vi "MPU_Stick_UI_Event_Handler.vi"(8 "error in (no error)":errorcluster, 11 "MPU_Stick_Globals":T3) -> ()   [LabVIEW 2017]
uses:
  Controls/MPU_Stick_Globals.ctl
  Controls/IMU_Configuration_References.ctl
  Controls/MP_Comp_Filter_Constants_References.ctl
  Controls/MD_Threshold_References.ctl
  Controls/MD_Type_References.ctl
  Controls/LED_Configuration_References.ctl
  Controls/Primary_References.ctl
  Controls/MPU_Stick_Queues.ctl
  Controls/MPU_Stick_Queue_Element.ctl
  Controls/MPU_Stick_Queue_Commands.ctl
  Classes/ADCP.lvclass
  <vilib>/Utility/miscctls.llb/LVPointDoubleTypeDef.ctl
  Controls/MPU_Stick_Read_Write_Configurations_Command.ctl
  Controls/MPU_Stick_Config_Parameters.ctl
  Controls/MPU_Stick_Plotter_Core_Commands.ctl
  <vilib>/Utility/miscctls.llb/LVOffsetAndMultiplierTypeDef.ctl
  MPU_Stick_Read_Serial_Port_Emulator.vi
panel:
  out "Primary.Parameter to monitor A":T1(ring)
  out "Primary.Cursor Position":T2
  out "Primary.Parameter to monitor":T1(ring)
  out "Primary.Offset":dbl
  out "Primary.Gain":dbl
  out "Primary.Get Gain & Offset":bool
  out "Primary.Set Gain & Offset":bool
  out "Primary.Remove graph parameter":bool
  out "Primary.Add graph parameter":bool
  out "MD Types Config.Set Parameter Index":u32
  out "MD Types Config.Get Parameter Index":u32
  out "MD Thresholds Config.Get Parameter Index":u32
  out "MD Thresholds Config.Set Parameter Index":u32
  out "Filter constants Config.Set Parameter Index":u32
  out "Filter constants Config.Get Parameter Index":u32
  out "LED Config.Set Parameter Index":u32
  out "LED Config.Get Parameter Index":u32
  out "IMU Config.Set Parameter Index":u32
  out "IMU Config.Get Parameter Index":u32
  out "Primary.MP Reset":bool
  out "Primary.Calibrate Sensor":bool
  out "Primary.Save all config":bool
  out "Primary.Write all config":bool
  out "Primary.Read all config":bool
  out "Primary.Connect Device":bool
  out "Primary.Exit Application":bool
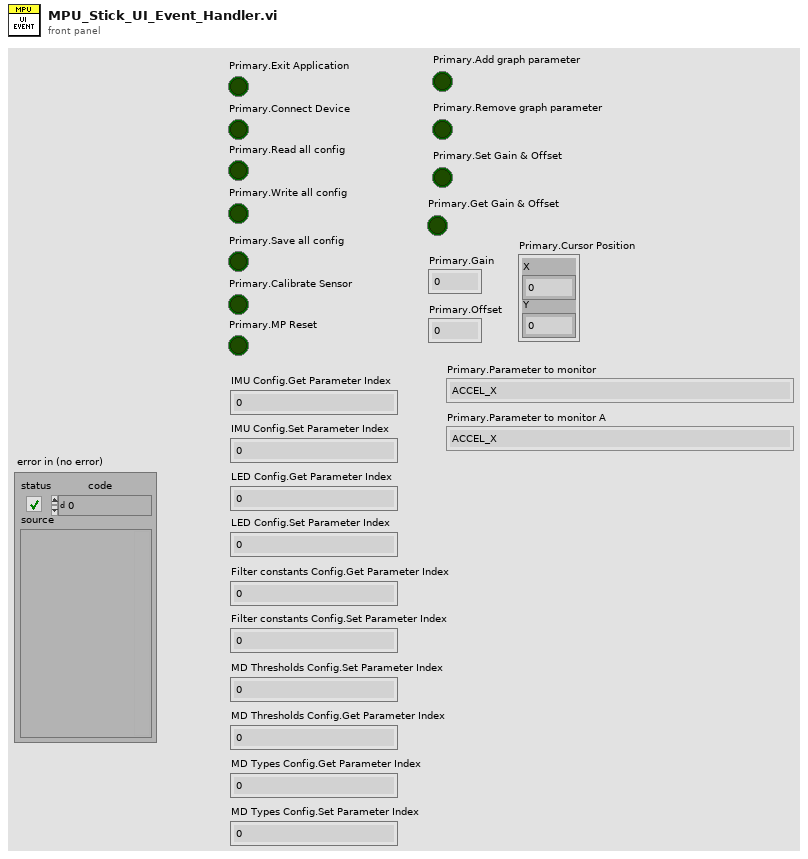
[diagram p1: front panel]
types:
  T1 = enum16{"ACCEL_X", "ACCEL_Y", "ACCEL_Z", "GYRO_X", "GYRO_Y", "GYRO_Z", "ROLL_ACCEL", "ROLL_GYRO", "ROLL_COMP_FILTER", "PITCH_ACCEL", "PITCH_GYRO", "PITCH_COMP_FILTER", "YAW_ACCEL", "YAW_GYRO", "YAW_COMP_FILTER"}
  T2 = typedef "LVPointDoubleTypeDef.ctl" = cluster{"X":dbl, "Y":dbl}
  T3 = typedef "MPU_Stick_Globals.ctl" = cluster{"IMU_configuration_references":T4, "MP_Comp_Filter_Constants_References":T5, "MD_Threshold_References":T6, "MD_Type_References":T7, "LED_Configuration_References":T8, "Primary_references":T9, "MPU_Stick_Queues":T10, "ADCP":refnum<vi>}
  T4 = typedef "IMU_Configuration_References.ctl" = cluster{"Get all IMU configurations":refnum<vi>, "Set all IMU configurations":refnum<vi>, "Get sampling frequency":refnum<vi>, "Set sampling frequency":refnum<vi>, "Get calibration point count":refnum<vi>, "Set calibration point count":refnum<vi>, "Get calibration interval":refnum<vi>, "Set calibration interval":refnum<vi>, "Get Gyroscope bandwidth":refnum<vi>, "Set Gyroscope bandwidth":refnum<vi>, "Get Gyroscope F.S. Value":refnum<vi>, "Set Gyroscope F.S. Value":refnum<vi>, "Get Accelerometer bandwidth":refnum<vi>, "Set Accelerometer bandwidth":refnum<vi>, "Get Accelerometer F.S. Value":refnum<vi>, "Set Accelerometer F.S. Value":refnum<vi>, "Sampling frequency (Hz)":refnum<vi>, "Calibration point count":refnum<vi>, "Calibration interval (ms)":refnum<vi>, "IMU Gyroscope bandwidth":refnum<vi>, "IMU Gyroscope F.S. value":refnum<vi>, "IMU Accelerometer bandwidth":refnum<vi>, "IMU Accelerometer F.S. value":refnum<vi>}
  T5 = typedef "MP_Comp_Filter_Constants_References.ctl" = cluster{"Set pitch filter constant":refnum<vi>, "Get pitch filter constant":refnum<vi>, "Set roll filter constant":refnum<vi>, "Get roll filter constant":refnum<vi>, "Pitch filter constant":refnum<vi>, "Roll filter constant":refnum<vi>}
  T6 = typedef "MD_Threshold_References.ctl" = cluster{"Yaw threshold (U)":refnum<vi>, "Yaw threshold (L)":refnum<vi>, "Pitch threshold (U)":refnum<vi>, "Pitch. threshold (L)":refnum<vi>, "Roll threshold (U)":refnum<vi>, "Roll threshold (L)":refnum<vi>, "Z gyro. threshold (U)":refnum<vi>, "Z gyro. threshold (L)":refnum<vi>, "Y gyro. threshold (U)":refnum<vi>, "Y gyro. threshold (L)":refnum<vi>, "X gyro. threshold (U)":refnum<vi>, "X gyro. threshold (L)":refnum<vi>, "Z accel. threshold (U)":refnum<vi>, "Z accel. threshold (L)":refnum<vi>, "Y accel. threshold (U)":refnum<vi>, "Y accel. threshold (L)":refnum<vi>, "X accel. threshold (U)":refnum<vi>, "X accel. threshold (L)":refnum<vi>, "Set all Motion detection threshold configurations":refnum<vi>, "Get yaw threshold (upper)":refnum<vi>, "Get yaw threshold (lower)":refnum<vi>, "Get pitch threshold (upper)":refnum<vi>, "Get pitch threshold (lower)":refnum<vi>, "Get roll threshold (upper)":refnum<vi>, "Get roll threshold (lower)":refnum<vi>, "Get Z gyro threshold (upper)":refnum<vi>, "Get Z gyro threshold (lower)":refnum<vi>, "Get Y gyro threshold (upper)":refnum<vi>, "Get Y gyro threshold (lower)":refnum<vi>, "Get X gyro threshold (upper)":refnum<vi>, "Get X gyro threshold (lower)":refnum<vi>, "Get Z accel threshold (upper)":refnum<vi>, "Get Z accel threshold (lower)":refnum<vi>, "Get Y accel threshold (upper)":refnum<vi>, "Get Y accel threshold (lower)":refnum<vi>, "Get X accel threshold (upper)":refnum<vi>, "Get X accel threshold (lower)":refnum<vi>, "Get all Motion detection threshold configurations":refnum<vi>, "Set yaw threshold (upper)":refnum<vi>, "Set yaw threshold (lower)":refnum<vi>, "Set pitch threshold (upper)":refnum<vi>, "Set pitch threshold (lower)":refnum<vi>, "Set roll threshold (upper)":refnum<vi>, "Set roll threshold (lower)":refnum<vi>, "Set Z gyro threshold (upper)":refnum<vi>, "Set Z gyro threshold (lower)":refnum<vi>, "Set Y gyro threshold (upper)":refnum<vi>, "Set Y gyro threshold (lower)":refnum<vi>, "Set X gyro threshold (upper)":refnum<vi>, "Set X gyro threshold (lower)":refnum<vi>, "Set Z accel threshold (upper)":refnum<vi>, "Set Z accel threshold (lower)":refnum<vi>, "Set Y accel threshold (upper)":refnum<vi>, "Set Y accel threshold (lower)":refnum<vi>, "Set X accel threshold (upper)":refnum<vi>, "Set X accel threshold (lower)":refnum<vi>}
  T7 = typedef "MD_Type_References.ctl" = cluster{"Yaw threshold type":refnum<vi>, "Pitch threshold type":refnum<vi>, "Roll threshold type":refnum<vi>, "Z gyro threshold type":refnum<vi>, "Y gyro threshold type":refnum<vi>, "X gyro threshold type":refnum<vi>, "Z accel threshold type":refnum<vi>, "Y accel threshold type":refnum<vi>, "X accel threshold type":refnum<vi>, "Set all Motion detection type configurations":refnum<vi>, "Get all Motion detection type configurations":refnum<vi>, "Set yaw threshold type":refnum<vi>, "Get yaw threshold type":refnum<vi>, "Set pitch threshold type":refnum<vi>, "Get pitch threshold type":refnum<vi>, "Set roll threshold type":refnum<vi>, "Get roll threshold type":refnum<vi>, "Set Z gyroscope threshold type":refnum<vi>, "Get Z gyroscope threshold type":refnum<vi>, "Set Y gyroscope threshold type":refnum<vi>, "Get Y gyroscope threshold type":refnum<vi>, "Set X gyroscope threshold type":refnum<vi>, "Get X gyroscope threshold type":refnum<vi>, "Set Z accel threshold type":refnum<vi>, "Get Z accel threshold type":refnum<vi>, "Set Y accel threshold type":refnum<vi>, "Get Y accel threshold type":refnum<vi>, "Get X accel threshold type":refnum<vi>, "Set X accel threshold type":refnum<vi>}
  T8 = typedef "LED_Configuration_References.ctl" = cluster{"Get all LED configurations":refnum<vi>, "Set all LED configurations":refnum<vi>, "Get LED3 configuration":refnum<vi>, "Set LED3 configuration":refnum<vi>, "Get LED2 configuration":refnum<vi>, "Set LED2 configuration":refnum<vi>, "Get LED1 configuration":refnum<vi>, "Set LED1 configuration":refnum<vi>, "LED3 Configuration":refnum<vi>, "LED2 Configuration":refnum<vi>, "LED1 Configuration":refnum<vi>}
  T9 = typedef "Primary_References.ctl" = cluster{"3D View Image":refnum<vi>, "Plot":refnum<vi>, "Graph / 3D view tab control":refnum<vi>, "MP Reset":refnum<vi>, "Calibrate IMU":refnum<vi>, "Plot Parameter List":refnum<vi>, "Remove Parameter from Plot":refnum<vi>, "Add Parameter to Plot":refnum<vi>, "Parameter to monitor":refnum<vi>, "Yaw motion detection output":refnum<vi>, "Pitch motion detection output":refnum<vi>, "Roll motion detection output":refnum<vi>, "Z gyro motion detection output":refnum<vi>, "Y gyro motion detection output":refnum<vi>, "X gyro motion detection output":refnum<vi>, "Z accel motion detection output":refnum<vi>, "Y accel motion detection output":refnum<vi>, "X accel motion detection output":refnum<vi>, "Yaw angle (filter) (degrees)":refnum<vi>, "Pitch angle (filter) (degrees)":refnum<vi>, "Roll angle (filter) (degrees)":refnum<vi>, "Yaw angle (gyro) (degrees)":refnum<vi>, "Pitch angle (gyro) (degrees)":refnum<vi>, "Roll angle (gyro) (degrees)":refnum<vi>, "Yaw angle (accel) (degrees)":refnum<vi>, "Pitch angle (accel) (degrees)":refnum<vi>, "Roll angle (accel) (degrees)":refnum<vi>, "Z gyroscope reading (DPS)":refnum<vi>, "Y gyroscope reading (DPS)":refnum<vi>, "X gyroscope reading (DPS)":refnum<vi>, "Z accelerometer reading (G)":refnum<vi>, "Y accelerometer reading (G)":refnum<vi>, "X accelerometer reading (G)":refnum<vi>, "Save all config.":refnum<vi>, "Write all config.":refnum<vi>, "Read all config.":refnum<vi>, "Tab Control":refnum<vi>, "Baud Rate":refnum<vi>, "COM Port":refnum<vi>, "Time (ms)":refnum<vi>, "Value (Units)":refnum<vi>, "Exit Application":refnum<vi>, "Connect Device":refnum<vi>, "Progress Bar":refnum<vi>, "Get Range & Offset":refnum<vi>, "Range":refnum<vi>, "Offset":refnum<vi>, "Set Range & Offset":refnum<vi>, "Parameter name":refnum<vi>, "Plot time (ms)":refnum<vi>, "Plot value":refnum<vi>}
  T10 = typedef "MPU_Stick_Queues.ctl" = cluster{"UI Event Handler":refnum<queue>, "3D View Updater":refnum<queue>, "Plot Updater":refnum<queue>, "Serial Port Reader":refnum<queue>, "UI Indicators Updater":refnum<queue>}
  T11 = typedef "MPU_Stick_Queue_Element.ctl" = cluster{"Data":variant, "Command":T12}
  T12 = typedef "MPU_Stick_Queue_Commands.ctl" = enum16{"UI_Event_Exit_Application_RQST", "UI_Event_Exit_Application_ACK", "UI_Event_Connect_Device_RQST", "UI_Event_Connect_Device_ACK", "UI_Event_Disconnect_Device_RQST", "UI_Event_Disconnect_Device_ACK", "UI_Event_Read_All_Configurations_RQST", "UI_Event_Read_All_Configurations_ACK", "UI_Event_Write_All_Configurations_RQST", "UI_Event_Write_All_Configurations_ACK", "UI_Event_Save_All_Configurations_RQST", "UI_Event_Save_All_Configurations_ACK", "UI_Event_Calibrate_IMU_Sensor_RQST", "UI_Event_Calibrate_IMU_Sensor_ACK", "UI_Event_MP_Reset_RQST", "UI_Event_MP_Reset_ACK", "UI_Event_Get_Config_RQST", "UI_Event_Get_Config_ACK", "UI_Event_Set_Config_RQST", "UI_Event_Set_Config_ACK", "Read_Serial_Port_Data_Pause", "Read_Serial_Port_Data_Pause_ACK", "Read_Serial_Port_Data_Continue", "Read_Serial_Port_Data_Exit", "Plotter_Exit", "Plotter_Update", "Plotter_Add_Channel", "Plotter_Remove_Channel", "3D Viewer Update", "3D Viewer Exit", "UI Indicators Update", "UI Indicators Exit"}
  T13 = typedef "MPU_Stick_Plotter_Core_Commands.ctl" = enum16{"Initialize", "Add Channel", "Remove Channel", "Set Channel Minimum Value", "Set Channel Maximum Value", "Set Offset & Multiplier", "Get Offset & Multiplier", "Update Channel", "Get Cursor Data", "Clear", "Reset"}
  T14 = typedef "LVOffsetAndMultiplierTypeDef.ctl" = cluster{"Offset":dbl, "Multiplier":dbl}
  T15 = typedef "MPU_Stick_Config_Parameters.ctl" = enum16{"IMU_ACCEL_FS", "IMU_ACCEL_BW", "IMU_GYRO_FS", "IMU_GYRO_BW", "IMU_CALIB_INTERVAL", "IMU_CALIB_POINT_COUNT", "IMU_SAMPLING_FREQ", "LED1_CONFIG", "LED2_CONFIG", "LED3_CONFIG", "MP_ROLL_FILTER_CONSTANT", "MP_PITCH_FILTER_CONSTANT", "MP_THRESHOLD_X_ACCEL_LOW", "MP_THRESHOLD_X_ACCEL_HIGH", "MP_THRESHOLD_Y_ACCEL_LOW", "MP_THRESHOLD_Y_ACCEL_HIGH", "MP_THRESHOLD_Z_ACCEL_LOW", "MP_THRESHOLD_Z_ACCEL_HIGH", "MP_THRESHOLD_X_GYRO_LOW", "MP_THRESHOLD_X_GYRO_HIGH", "MP_THRESHOLD_Y_GYRO_LOW", "MP_THRESHOLD_Y_GYRO_HIGH", "MP_THRESHOLD_Z_GYRO_LOW", "MP_THRESHOLD_Z_GYRO_HIGH", "MP_THRESHOLD_ROLL_LOW", "MP_THRESHOLD_ROLL_HIGH", "MP_THRESHOLD_PITCH_LOW", "MP_THRESHOLD_PITCH_HIGH", "MP_THRESHOLD_YAW_LOW", "MP_THRESHOLD_YAW_HIGH", "MP_DETECTION_TYPE_X_ACCEL", "MP_DETECTION_TYPE_Y_ACCEL", "MP_DETECTION_TYPE_Z_ACCEL", "MP_DETECTION_TYPE_X_GYRO", "MP_DETECTION_TYPE_Y_GYRO", "MP_DETECTION_TYPE_Z_GYRO", "MP_DETECTION_TYPE_ROLL", "MP_DETECTION_TYPE_PITCH", "MP_DETECTION_TYPE_YAW"}
  T16 = typedef "MPU_Stick_Plotter_Core_Channel_Data.ctl" = cluster{"Value (original)":dbl[], "Time (ms)":dbl[], "Channel name":string, "Minimum":dbl, "Maximum":dbl, "Offset":dbl, "Range":dbl}
  T17 = cluster{"Symbol File Path":path, "Transmit Log File Path":path, "Receive Log File Path":path, "COM Port":refnum<visa-resource-name>, "Baud rate":u32, "Number of retries":u16, "Retry interval (ms)":u16, "Session start time (ms)":u32, "Current time (ms)":u32, "Serialport timeout (ms)":u32}
  T18 = typedef "MPU_Stick_Read_Write_Configurations_Command.ctl" = enum16{"Read", "Write", "Write All", "Read All"}
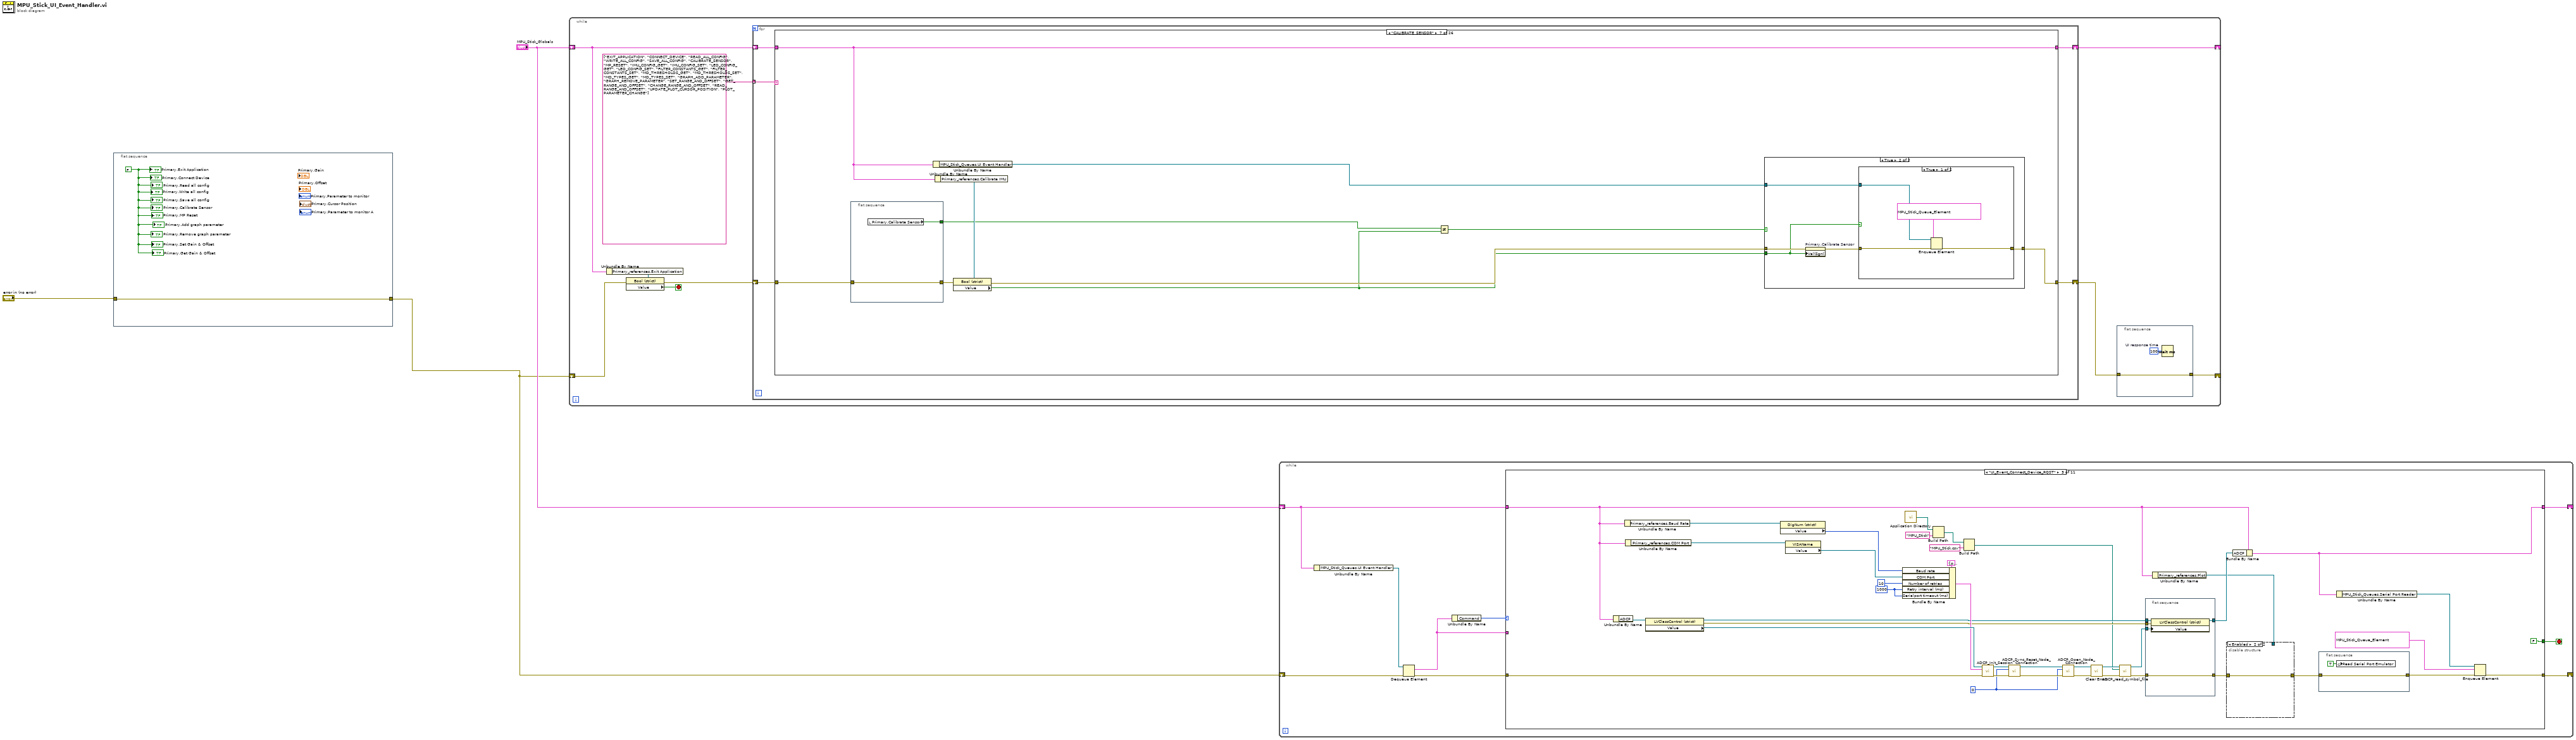
[diagram p0: block diagram]
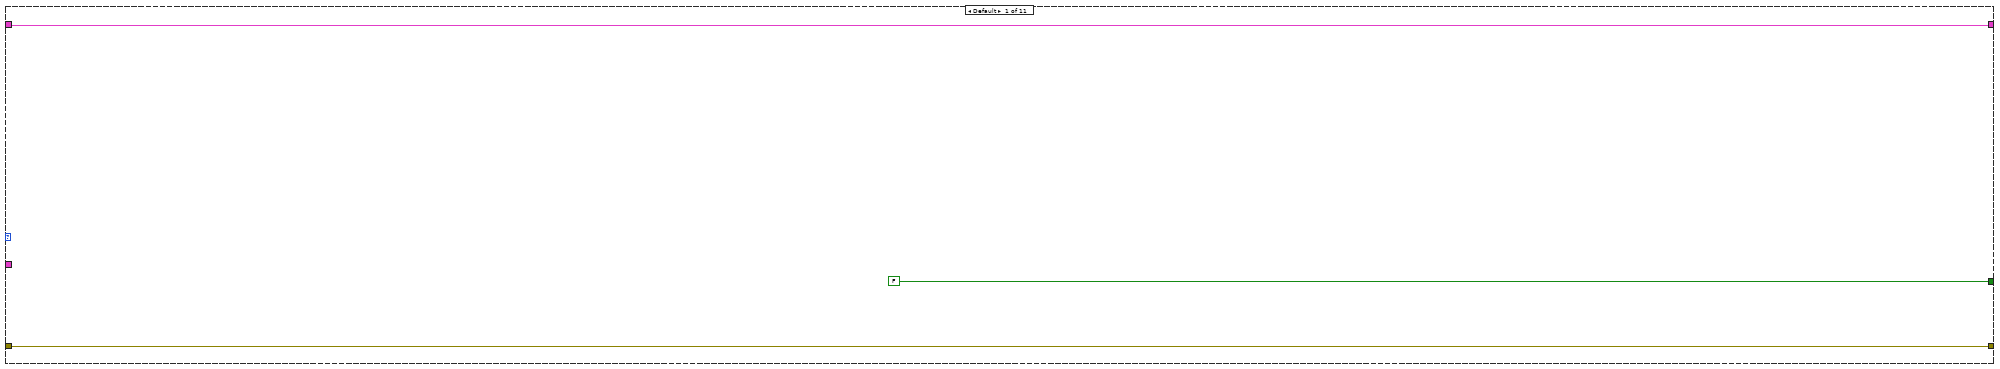
[diagram p2: hidden frame]
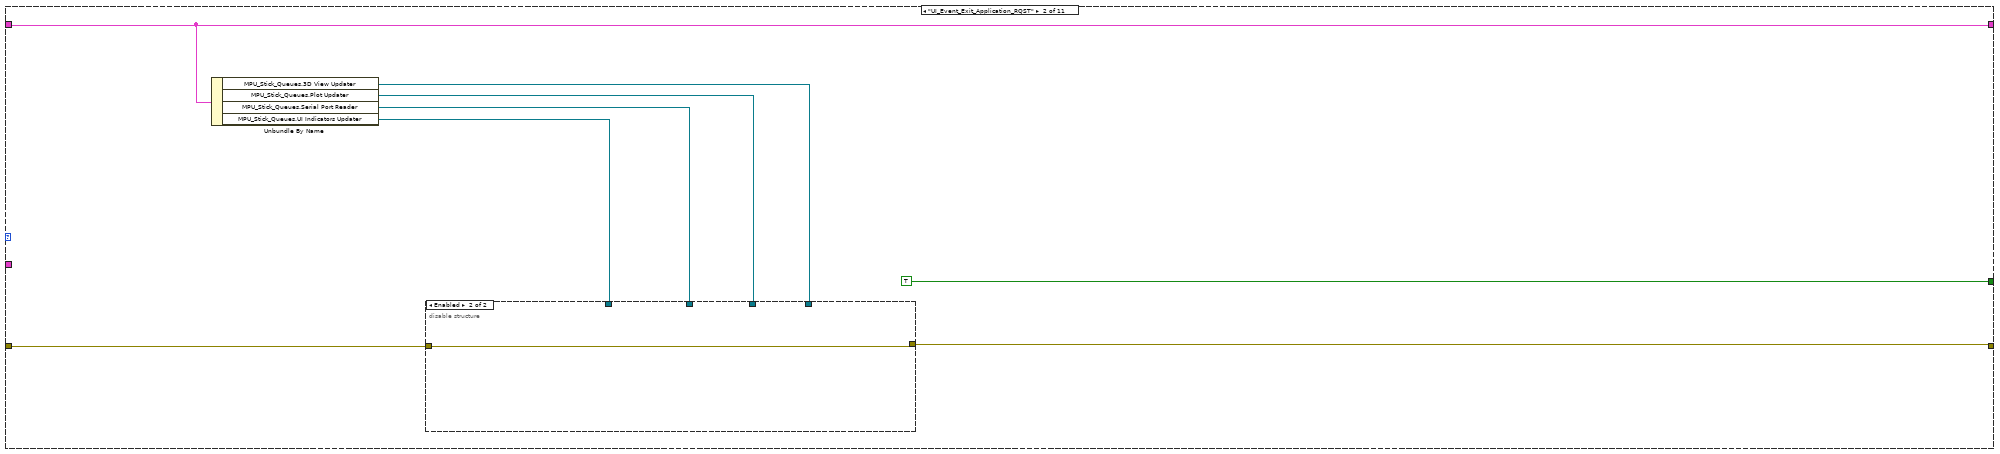
[diagram p3: hidden frame]
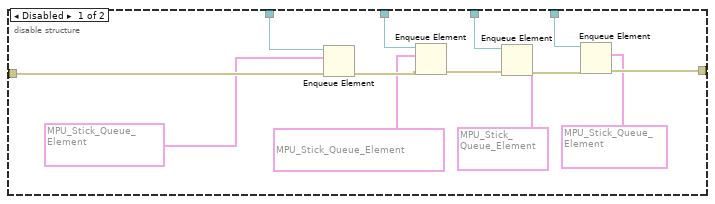
[diagram p4: hidden frame]
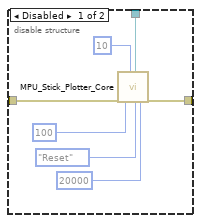
[diagram p5: hidden frame]
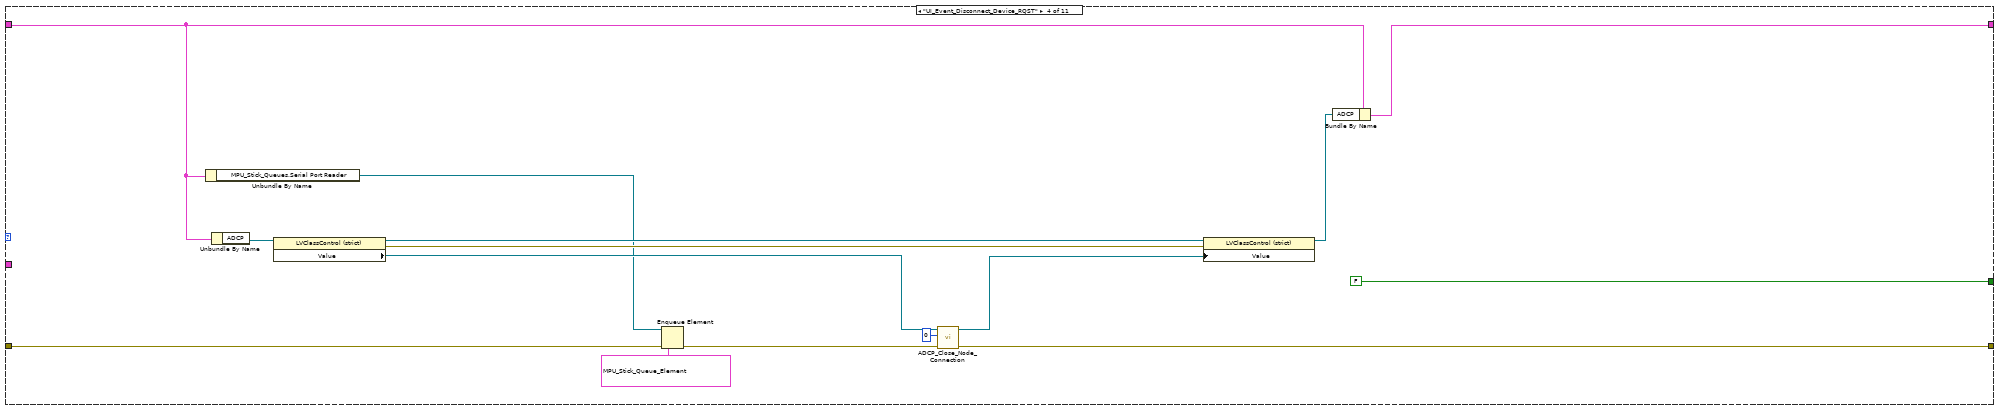
[diagram p6: hidden frame]
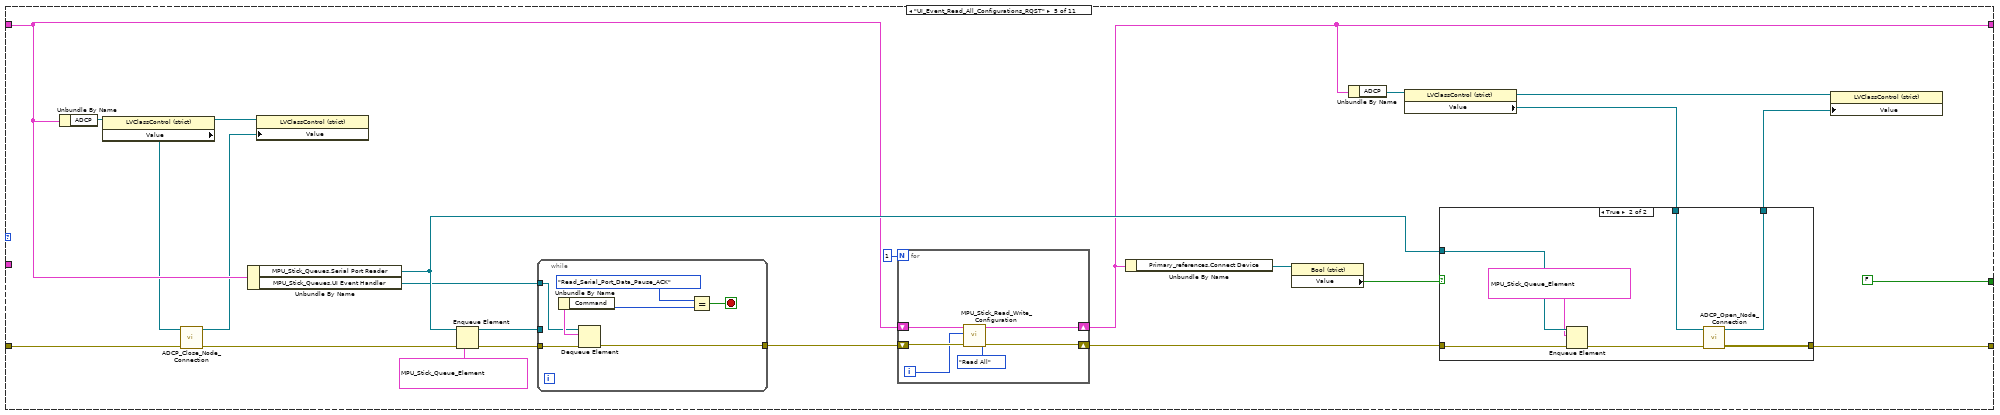
[diagram p7: hidden frame]
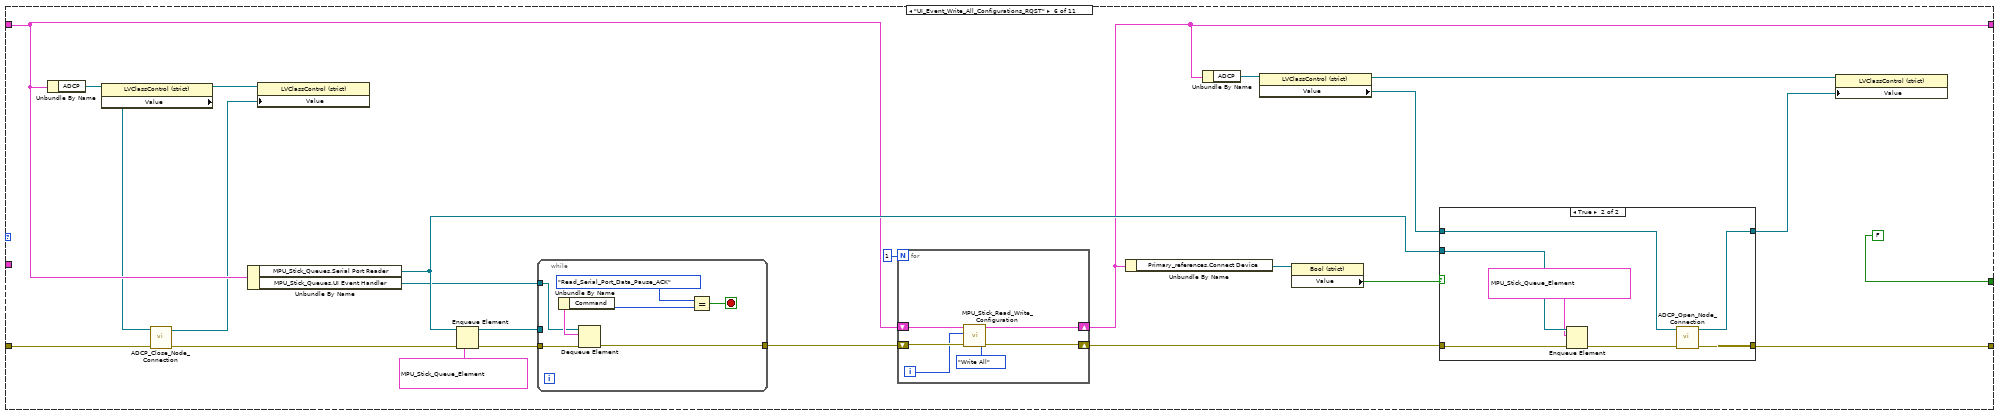
[diagram p9: hidden frame]
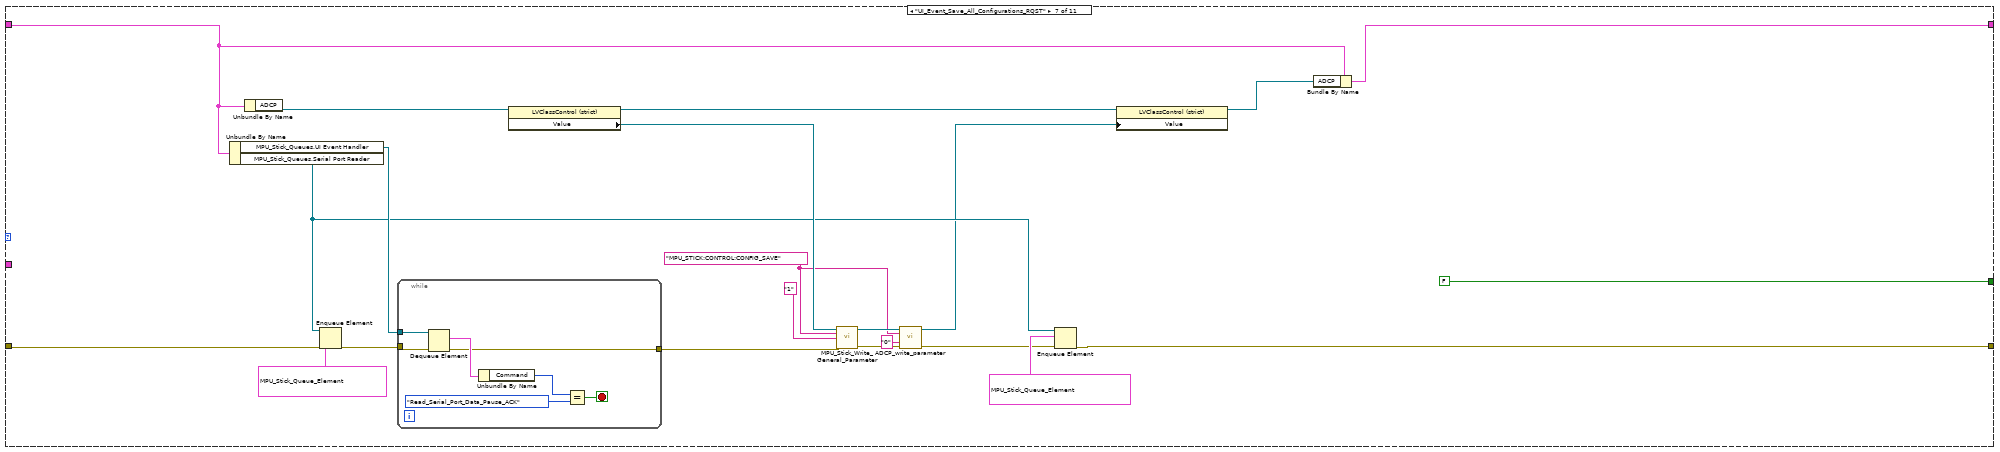
[diagram p11: hidden frame]
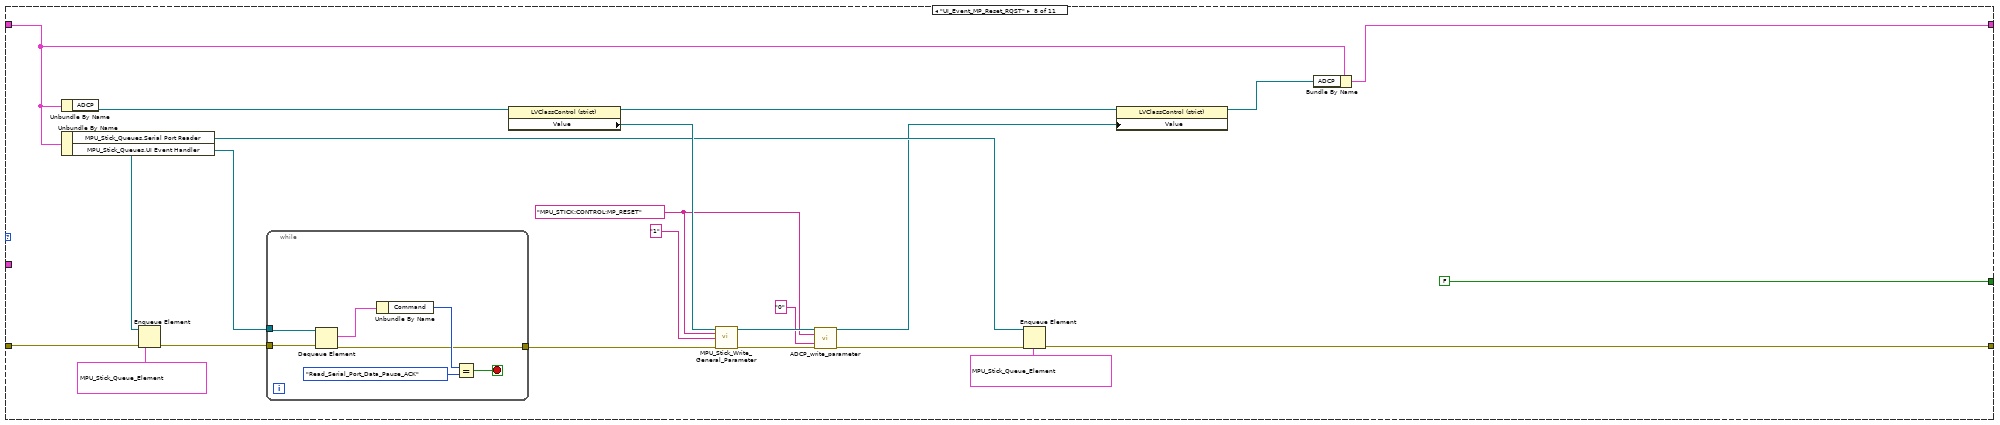
[diagram p12: hidden frame]
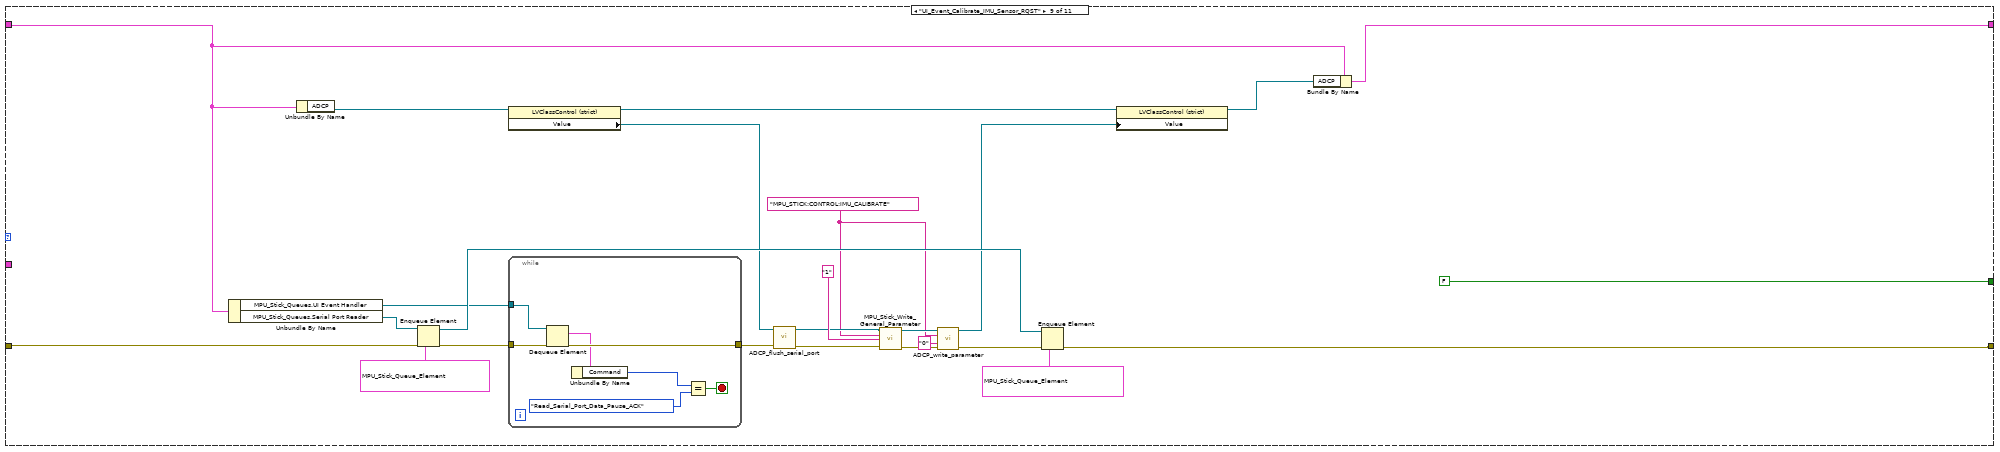
[diagram p13: hidden frame]
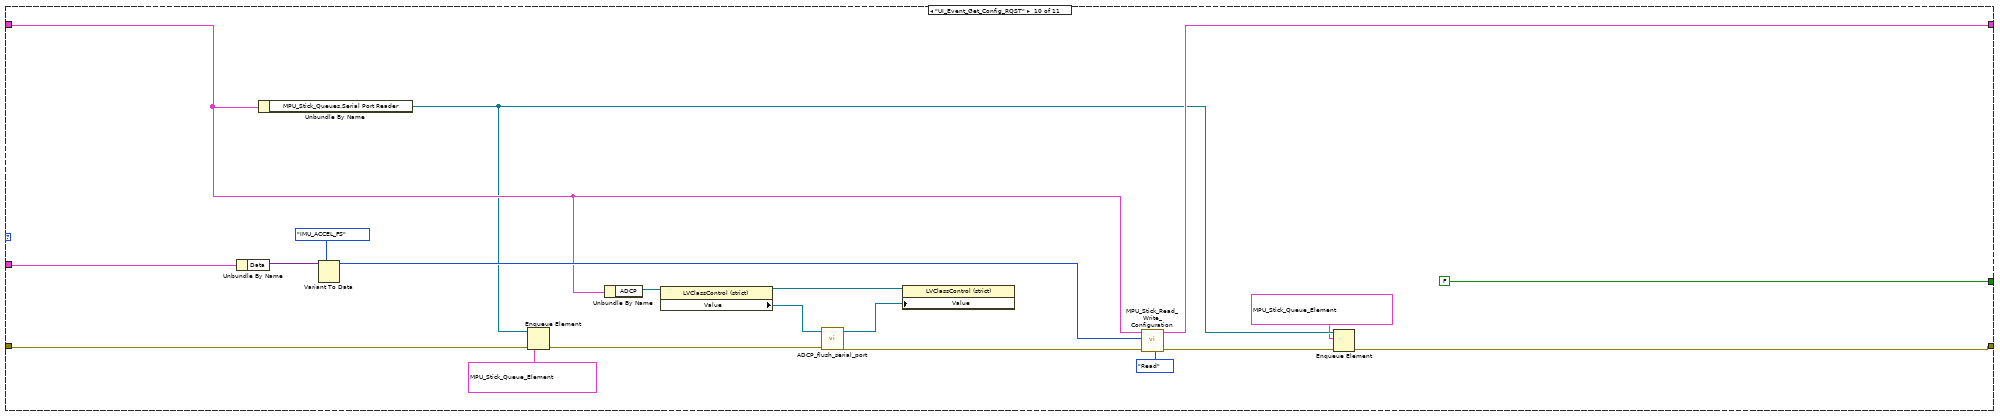
[diagram p14: hidden frame]
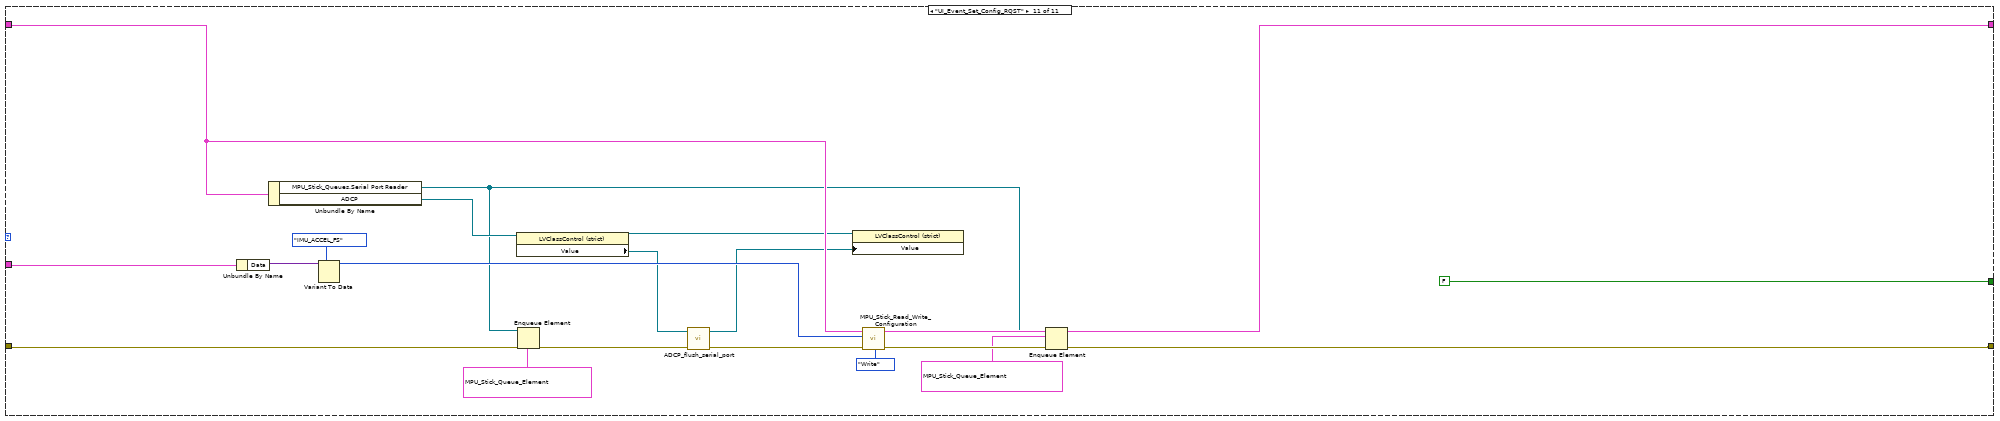
[diagram p15: hidden frame]
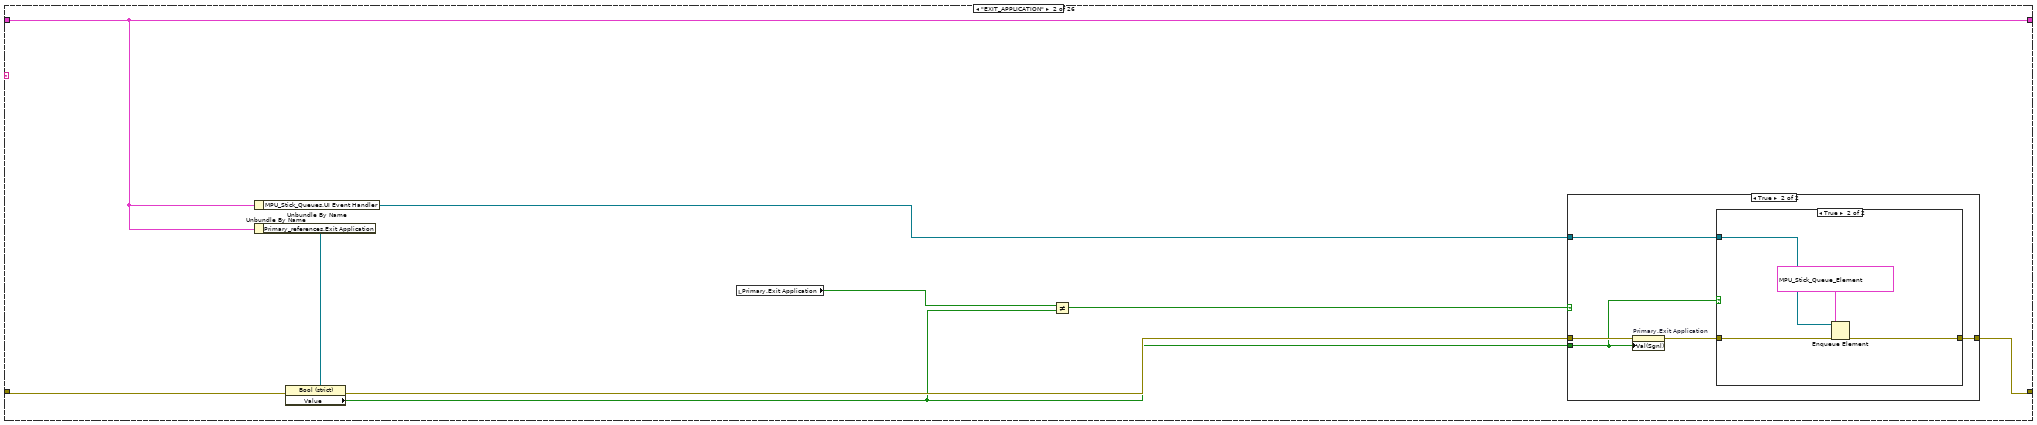
[diagram p17: hidden frame]
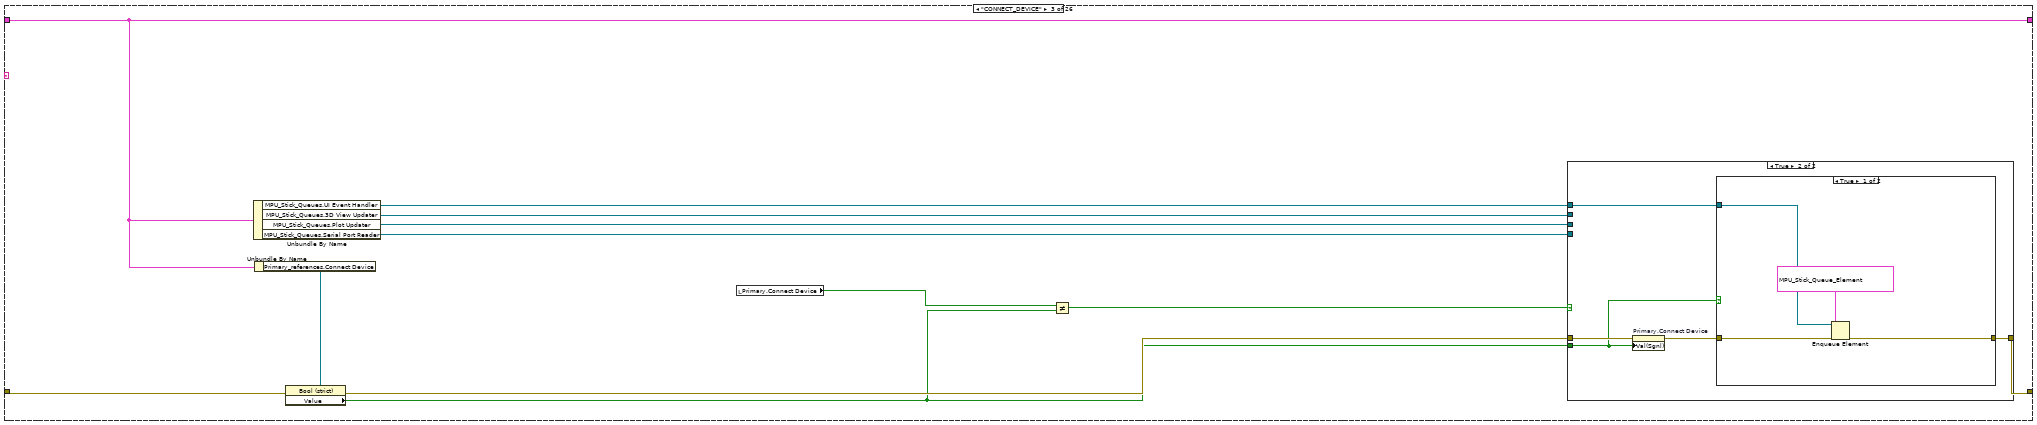
[diagram p20: hidden frame]
diagram:
  n1 = flat-sequence {
    tunnel: "error in (no error)" -> [w5]
    tunnel: [w5] -> w1
    frame #0 {
      w4 = FALSE ("Exit Application")
      "Primary.Exit Application" <- w4
      "Primary.Connect Device" <- w4
      "Primary.Read all config" <- w4
      "Primary.Write all config" <- w4
      "Primary.Save all config" <- w4
      "Primary.Calibrate Sensor" <- w4
      "Primary.MP Reset" <- w4
      "Primary.Add graph parameter" <- w4
      "Primary.Remove graph parameter" <- w4
      "Primary.Set Gain & Offset" <- w4
      "Primary.Get Gain & Offset" <- w4
    }
  }
  n2 = while {
    shift-right: [w10] -> _
    shift-left: "MPU_Stick_Globals" -> [w11]
    shift-right: [w6] -> _
    shift-left: w1 -> [w12]
    stop <- w13 stop-if-true
    n3 = Unbundle By Name(w11) -> ("Primary_references.Exit Application"=w14:refnum<vi>)
    n4 = property class="Bool (strict)"(reference=w14, error in=w12) -> (error out=w9:errorcluster, "Value"=w13:bool)  [unwired: 1 out]
    n5 = for {
      shift-right: [w18] -> w10
      shift-left: w11 -> [w19]
      shift-right: [w17] -> w7
      shift-left: w9 -> [w21]
      tunnel: string[] ["EXIT_APPLICATION", "CONNECT_DEVICE", "READ_ALL_CONFIG", "WRITE_ALL_CONFIG", "SAVE_ALL_CONFIG", "CALIBRATE_SENSOR", "MP_RESET", "IMU_CONFIG_GET", "IMU_CONFIG_SET", "LED_CONFIG_GET", "LED_CONFIG_SET", "FILTER_CONSTANTS_GET", "FILTER_CONSTANTS_SET", "MD_THRESHOLDS_GET", "MD_THRESHOLDS_SET", "MD_TYPES_GET", "MD_TYPES_SET", "GRAPH_ADD_PARAMETER", "GRAPH_REMOVE_PARAMETER", "SET_RANGE_AND_OFFSET", "GET_RANGE_AND_OFFSET", "CHANGE_RANGE_AND_OFFSET", "READ_RANGE_AND_OFFSET", "UPDATE_PLOT_CURSOR_POSITION", "PLOT_PARAMETER_CHANGE"] -> [w20] mode=indexing
      n6 = case shown="\"CALIBRATE_SENSOR\"" w20 {
        tunnel: w21 -> [w22 w31 w54 w77 w97 w117 w131 w160 w183 w243 w307 w363 w417 w471 w542 w613 w676 w738 w789 w831 w872 w916 w960 w1004 w1048 w1095]
        tunnel: w19 -> [w23 w25 w48 w71 w91 w111 w133 w154 w194 w254 w297 w353 w407 w461 w532 w603 w666 w728 w780 w822 w863 w907 w956 w1000 w1045 w1091]
        tunnel: [w23 w25 w48 w71 w91 w111 w133 w154 w194 w254 w297 w353 w407 w461 w532 w603 w666 w728 w780 w822 w863 w907 w956 w1000 w1045 w1091] -> w18
        tunnel: [w22 w29 w52 w75 w95 w115 w137 w158 w184 w244 w308 w364 w418 w472 w543 w614 w677 w739 w783 w825 w866 w910 w959 w1003 w1047 w1094] -> w17
        frame Default {
        }
        frame "EXIT_APPLICATION" {
          n7 = Unbundle By Name(w25) -> ("Primary_references.Exit Application"=w32:refnum<vi>)
          n8 = Unbundle By Name(w25) -> ("MPU_Stick_Queues.UI Event Handler"=w24:refnum<queue>)
          n9 = property class="Bool (strict)"(reference=w32, error in=w31) -> (error out=w30:errorcluster, "Value"=w26:bool)  [unwired: 1 out]
          n10 = local read "Primary.Exit Application"() -> (w28:bool)
          n11 = Not Equal?(x=w28, y=w26) -> (x != y?=w27:bool)
          n12 = case shown="True" w27 {
            tunnel: w30 -> [w33 w38]
            tunnel: [w33 w35] -> w29
            tunnel: w26 -> [_ w37]
            tunnel: w24 -> [_ w34]
            frame False {
            }
            frame True {
              n13 = property on="Primary.Exit Application" class="Bool (strict)"(error in=w38, "Val(Sgnl)"=w37) -> (error out=w36:errorcluster)  [unwired: 1 in, 1 out]
              n14 = case shown="True" w37 {
                tunnel: w36 -> [w39 w43]
                tunnel: [w39 w42] -> w35
                tunnel: w34 -> [_ w41]
                frame False {
                }
                frame True {
                  n15 = Enqueue Element(queue=w41, element=T11 {"Data"=variant, "Command"=enum."UI_Event_Exit_Application_RQST"}, error in (no error)=w43) -> (error out=w42:errorcluster)  [unwired: 1 in, 2 out]
                }
              }
            }
          }
        }
        frame "CONNECT_DEVICE" {
          n16 = Unbundle By Name(w48) -> ("MPU_Stick_Queues.UI Event Handler"=w47:refnum<queue>, "MPU_Stick_Queues.3D View Updater"=w46:refnum<queue>, "MPU_Stick_Queues.Plot Updater"=w45:refnum<queue>, "MPU_Stick_Queues.Serial Port Reader"=w44:refnum<queue>)
          n17 = Unbundle By Name(w48) -> ("Primary_references.Connect Device"=w55:refnum<vi>)
          n18 = property class="Bool (strict)"(reference=w55, error in=w54) -> (error out=w53:errorcluster, "Value"=w49:bool)  [unwired: 1 out]
          n19 = local read "Primary.Connect Device"() -> (w51:bool)
          n20 = Not Equal?(x=w51, y=w49) -> (x != y?=w50:bool)
          n21 = case shown="True" w50 {
            tunnel: w53 -> [w56 w61]
            tunnel: [w56 w58] -> w52
            tunnel: w49 -> [_ w60]
            tunnel: w47 -> [_ w57]
            tunnel: w46 -> [_ _]
            tunnel: w45 -> [_ _]
            tunnel: w44 -> [_ _]
            frame False {
            }
            frame True {
              n22 = property on="Primary.Connect Device" class="Bool (strict)"(error in=w61, "Val(Sgnl)"=w60) -> (error out=w59:errorcluster)  [unwired: 1 in, 1 out]
              n23 = case shown="True" w60 {
                tunnel: w59 -> [w65 w69]
                tunnel: [w64 w68] -> w58
                tunnel: w57 -> [w63 w67]
                frame True {
                  n24 = Enqueue Element(queue=w63, element=T11 {"Data"=variant, "Command"=enum."UI_Event_Connect_Device_RQST"}, error in (no error)=w65) -> (error out=w64:errorcluster)  [unwired: 1 in, 2 out]
                }
                frame False {
                  n25 = Enqueue Element(queue=w67, element=T11 {"Data"=variant, "Command"=enum."UI_Event_Disconnect_Device_RQST"}, error in (no error)=w69) -> (error out=w68:errorcluster)  [unwired: 1 in, 2 out]
                }
              }
            }
          }
        }
        frame "READ_ALL_CONFIG" {
          n26 = Unbundle By Name(w71) -> ("MPU_Stick_Queues.UI Event Handler"=w70:refnum<queue>)
          n27 = Unbundle By Name(w71) -> ("Primary_references.Read all config."=w78:refnum<vi>)
          n28 = property class="Bool (strict)"(reference=w78, error in=w77) -> (error out=w76:errorcluster, "Value"=w72:bool)  [unwired: 1 out]
          n29 = local read "Primary.Read all config"() -> (w74:bool)
          n30 = Not Equal?(x=w74, y=w72) -> (x != y?=w73:bool)
          n31 = case shown="True" w73 {
            tunnel: w76 -> [w79 w84]
            tunnel: [w79 w81] -> w75
            tunnel: w72 -> [_ w83]
            tunnel: w70 -> [_ w80]
            frame False {
            }
            frame True {
              n32 = property on="Primary.Read all config" class="Bool (strict)"(error in=w84, "Val(Sgnl)"=w83) -> (error out=w82:errorcluster)  [unwired: 1 in, 1 out]
              n33 = case shown="False" w83 {
                tunnel: w82 -> [w88 w89]
                tunnel: [w87 w89] -> w81
                tunnel: w80 -> [w86 _]
                frame True {
                  n34 = Enqueue Element(queue=w86, element=T11 {"Data"=variant, "Command"=enum."UI_Event_Read_All_Configurations_RQST"}, error in (no error)=w88) -> (error out=w87:errorcluster)  [unwired: 1 in, 2 out]
                }
                frame False {
                }
              }
            }
          }
        }
        frame "WRITE_ALL_CONFIG" {
          n35 = Unbundle By Name(w91) -> ("Primary_references.Write all config."=w98:refnum<vi>)
          n36 = Unbundle By Name(w91) -> ("MPU_Stick_Queues.UI Event Handler"=w90:refnum<queue>)
          n37 = property class="Bool (strict)"(reference=w98, error in=w97) -> (error out=w96:errorcluster, "Value"=w92:bool)  [unwired: 1 out]
          n38 = local read "Primary.Write all config"() -> (w94:bool)
          n39 = Not Equal?(x=w94, y=w92) -> (x != y?=w93:bool)
          n40 = case shown="True" w93 {
            tunnel: w96 -> [w99 w104]
            tunnel: [w99 w101] -> w95
            tunnel: w92 -> [_ w103]
            tunnel: w90 -> [_ w100]
            frame False {
            }
            frame True {
              n41 = property on="Primary.Write all config" class="Bool (strict)"(error in=w104, "Val(Sgnl)"=w103) -> (error out=w102:errorcluster)  [unwired: 1 in, 1 out]
              n42 = case shown="True" w103 {
                tunnel: w102 -> [w108 w109]
                tunnel: [w107 w109] -> w101
                tunnel: w100 -> [w106 _]
                frame True {
                  n43 = Enqueue Element(queue=w106, element=T11 {"Data"=variant, "Command"=enum."UI_Event_Write_All_Configurations_RQST"}, error in (no error)=w108) -> (error out=w107:errorcluster)  [unwired: 1 in, 2 out]
                }
                frame False {
                }
              }
            }
          }
        }
        frame "SAVE_ALL_CONFIG" {
          n44 = Unbundle By Name(w111) -> ("MPU_Stick_Queues.UI Event Handler"=w110:refnum<queue>)
          n45 = Unbundle By Name(w111) -> ("Primary_references.Save all config."=w118:refnum<vi>)
          n46 = property class="Bool (strict)"(reference=w118, error in=w117) -> (error out=w116:errorcluster, "Value"=w112:bool)  [unwired: 1 out]
          n47 = local read "Primary.Save all config"() -> (w114:bool)
          n48 = Not Equal?(x=w114, y=w112) -> (x != y?=w113:bool)
          n49 = case shown="True" w113 {
            tunnel: w116 -> [w119 w124]
            tunnel: [w119 w121] -> w115
            tunnel: w112 -> [_ w123]
            tunnel: w110 -> [_ w120]
            frame False {
            }
            frame True {
              n50 = property on="Primary.Save all config" class="Bool (strict)"(error in=w124, "Val(Sgnl)"=w123) -> (error out=w122:errorcluster)  [unwired: 1 in, 1 out]
              n51 = case shown="True" w123 {
                tunnel: w122 -> [w128 w129]
                tunnel: [w127 w129] -> w121
                tunnel: w120 -> [w126 _]
                frame True {
                  n52 = Enqueue Element(queue=w126, element=T11 {"Data"=variant, "Command"=enum."UI_Event_Save_All_Configurations_RQST"}, error in (no error)=w128) -> (error out=w127:errorcluster)  [unwired: 1 in, 2 out]
                }
                frame False {
                }
              }
            }
          }
        }
        frame "CALIBRATE_SENSOR" {
          n53 = flat-sequence {
            tunnel: [w141] -> w136
            tunnel: w131 -> [w140]
            tunnel: [w140] -> w130
            frame #0 {
              n54 = local read "Primary.Calibrate Sensor"() -> (w141:bool)
            }
          }
          n55 = Unbundle By Name(w133) -> ("MPU_Stick_Queues.UI Event Handler"=w132:refnum<queue>)
          n56 = Unbundle By Name(w133) -> ("Primary_references.Calibrate IMU"=w139:refnum<vi>)
          n57 = property class="Bool (strict)"(reference=w139, error in=w130) -> (error out=w138:errorcluster, "Value"=w134:bool)  [unwired: 1 out]
          n58 = Not Equal?(x=w136, y=w134) -> (x != y?=w135:bool)
          n59 = case shown="True" w135 {
            tunnel: w138 -> [w142 w147]
            tunnel: [w142 w144] -> w137
            tunnel: w134 -> [_ w146]
            tunnel: w132 -> [_ w143]
            frame False {
            }
            frame True {
              n60 = property on="Primary.Calibrate Sensor" class="Bool (strict)"(error in=w147, "Val(Sgnl)"=w146) -> (error out=w145:errorcluster)  [unwired: 1 in, 1 out]
              n61 = case shown="True" w146 {
                tunnel: w145 -> [w151 w152]
                tunnel: [w150 w152] -> w144
                tunnel: w143 -> [w149 _]
                frame True {
                  n62 = Enqueue Element(queue=w149, element=T11 {"Data"=variant, "Command"=enum."UI_Event_Calibrate_IMU_Sensor_RQST"}, error in (no error)=w151) -> (error out=w150:errorcluster)  [unwired: 1 in, 2 out]
                }
                frame False {
                }
              }
            }
          }
        }
        frame "MP_RESET" {
          n63 = Unbundle By Name(w154) -> ("MPU_Stick_Queues.UI Event Handler"=w153:refnum<queue>)
          n64 = Unbundle By Name(w154) -> ("Primary_references.MP Reset"=w161:refnum<vi>)
          n65 = property class="Bool (strict)"(reference=w161, error in=w160) -> (error out=w159:errorcluster, "Value"=w155:bool)  [unwired: 1 out]
          n66 = local read "Primary.MP Reset"() -> (w157:bool)
          n67 = Not Equal?(x=w157, y=w155) -> (x != y?=w156:bool)
          n68 = case shown="True" w156 {
            tunnel: w159 -> [w162 w167]
            tunnel: [w162 w164] -> w158
            tunnel: w155 -> [_ w166]
            tunnel: w153 -> [_ w163]
            frame False {
            }
            frame True {
              n69 = property on="Primary.MP Reset" class="Bool (strict)"(error in=w167, "Val(Sgnl)"=w166) -> (error out=w165:errorcluster)  [unwired: 1 in, 1 out]
              n70 = case shown="True" w166 {
                tunnel: w165 -> [w171 w172]
                tunnel: [w170 w172] -> w164
                tunnel: w163 -> [w169 _]
                frame True {
                  n71 = Enqueue Element(queue=w169, element=T11 {"Data"=variant, "Command"=enum."UI_Event_MP_Reset_RQST"}, error in (no error)=w171) -> (error out=w170:errorcluster)  [unwired: 1 in, 2 out]
                }
                frame False {
                }
              }
            }
          }
        }
        frame "IMU_CONFIG_GET" {
          n72 = Unbundle By Name(w194) -> ("MPU_Stick_Queues.UI Event Handler"=w193:refnum<queue>)
          n73 = Unbundle By Name(w194) -> ("IMU_configuration_references.Get Accelerometer F.S. Value"=w192:refnum<vi>, "IMU_configuration_references.Get Accelerometer bandwidth"=w191:refnum<vi>, "IMU_configuration_references.Get Gyroscope F.S. Value"=w190:refnum<vi>, "IMU_configuration_references.Get Gyroscope bandwidth"=w189:refnum<vi>, "IMU_configuration_references.Get calibration interval"=w188:refnum<vi>, "IMU_configuration_references.Get calibration point count"=w187:refnum<vi>, "IMU_configuration_references.Get sampling frequency"=w186:refnum<vi>, "IMU_configuration_references.Get all IMU configurations"=w178:refnum<vi>)
          n74 = flat-sequence {
            tunnel: w183 -> [w197]
            tunnel: [w197] -> w182
            tunnel: [w196] -> w179
            frame #0 {
              n75 = local read "IMU Config.Get Parameter Index"() -> (w196:u32)
            }
          }
          n76 = Build Array(w192, w191, w190, w189, w188, w187, w186, w178) -> (w185:refnum<vi>[])
          n77 = for {
            tunnel: w185 -> [w201] mode=indexing
            shift-right: [w200] -> w181
            shift-left: w182 -> [w202]
            tunnel: [w199] -> w177
            tunnel: [w198] -> w173
            i -> [w199]
            stop <- w198 stop-if-true
            n78 = property class="Bool (strict)"(reference=w201, error in=w202) -> (error out=w200:errorcluster, "Value"=w198:bool)  [unwired: 1 out]
          }
          n79 = Increment(x=w177) -> (x+1=w175:i32)
          n80 = Select(t=w175, s=w173, f=0) -> (s? t:f=w176:i32)
          n81 = To Unsigned Long Integer(number=w176) -> (unsigned 32bit integer=w180:u32)
          "IMU Config.Get Parameter Index" <- w180
          n82 = Not Equal?(x=w180, y=w179) -> (x != y?=w195:bool)
          n83 = case shown="True" w195 {
            tunnel: [w203 w209] -> w184
            tunnel: w193 -> [_ w208]
            tunnel: w181 -> [w203 w207]
            tunnel: w180 -> [_ w206]
            tunnel: w179 -> [_ w205]
            frame False {
            }
            frame True {
              w204 = T15[] [enum."IMU_ACCEL_FS", enum."IMU_ACCEL_BW", enum."IMU_GYRO_FS", enum."IMU_GYRO_BW", enum."IMU_CALIB_INTERVAL", enum."IMU_CALIB_POINT_COUNT", enum."IMU_SAMPLING_FREQ"] items=["IMU_ACCEL_FS", "IMU_ACCEL_BW", "IMU_GYRO_FS", "IMU_GYRO_BW", "IMU_CALIB_INTERVAL", "IMU_CALIB_POINT_COUNT", "IMU_SAMPLING_FREQ", "LED1_CONFIG", "LED2_CONFIG", "LED3_CONFIG", "MP_ROLL_FILTER_CONSTANT", "MP_PITCH_FILTER_CONSTANT", "MP_THRESHOLD_X_ACCEL_LOW", "MP_THRESHOLD_X_ACCEL_HIGH", "MP_THRESHOLD_Y_ACCEL_LOW", "MP_THRESHOLD_Y_ACCEL_HIGH", "MP_THRESHOLD_Z_ACCEL_LOW", "MP_THRESHOLD_Z_ACCEL_HIGH", "MP_THRESHOLD_X_GYRO_LOW", "MP_THRESHOLD_X_GYRO_HIGH", "MP_THRESHOLD_Y_GYRO_LOW", "MP_THRESHOLD_Y_GYRO_HIGH", "MP_THRESHOLD_Z_GYRO_LOW", "MP_THRESHOLD_Z_GYRO_HIGH", "MP_THRESHOLD_ROLL_LOW", "MP_THRESHOLD_ROLL_HIGH", "MP_THRESHOLD_PITCH_LOW", "MP_THRESHOLD_PITCH_HIGH", "MP_THRESHOLD_YAW_LOW", "MP_THRESHOLD_YAW_HIGH", "MP_DETECTION_TYPE_X_ACCEL", "MP_DETECTION_TYPE_Y_ACCEL", "MP_DETECTION_TYPE_Z_ACCEL", "MP_DETECTION_TYPE_X_GYRO", "MP_DETECTION_TYPE_Y_GYRO", "MP_DETECTION_TYPE_Z_GYRO", "MP_DETECTION_TYPE_ROLL", "MP_DETECTION_TYPE_PITCH", "MP_DETECTION_TYPE_YAW"]
              n84 = property on="IMU Config.Get Parameter Index" class="DigNum (strict)"(error in=w207, "Val(Sgnl)"=w206) -> (error out=w210:errorcluster)  [unwired: 1 in, 1 out]
              n85 = case shown="8" w205 {
                selector: w205 -> [w213 _ _]
                tunnel: w210 -> [w220 w224 w232]
                tunnel: [w219 w223 w232] -> w209
                tunnel: w208 -> [w218 w222 _]
                tunnel: w204 -> [w214 w221 _]
                frame 1..7 {
                  n86 = Decrement(x=w213) -> (x-1=w211:u32)
                  n87 = Index Array(array=w214, index=w211) -> (element=w212:T15)
                  n88 = To Variant(anything=w212) -> (Variant=w215:variant)
                  n89 = Bundle By Name(cluster=T11 {"Data"=variant, "Command"=enum."UI_Event_Get_Config_RQST"} ("element"), "Data"=w215) -> (w216:T11)
                  n90 = Enqueue Element(queue=w218, element=w216, error in (no error)=w220) -> (error out=w219:errorcluster)  [unwired: 1 in, 2 out]
                }
                frame 8 {
                  n91 = for {
                    tunnel: w222 -> [w229]
                    shift-right: [w230] -> w223
                    shift-left: w224 -> [w231]
                    tunnel: w221 -> [w225] mode=indexing
                    n92 = To Variant(anything=w225) -> (Variant=w226:variant)
                    n93 = Bundle By Name(cluster=T11 {"Data"=variant, "Command"=enum."UI_Event_Get_Config_RQST"} ("element"), "Data"=w226) -> (w227:T11)
                    n94 = Enqueue Element(queue=w229, element=w227, error in (no error)=w231) -> (error out=w230:errorcluster)  [unwired: 1 in, 2 out]
                  }
                }
                frame Default {
                }
              }
            }
          }
        }
        frame "IMU_CONFIG_SET" {
          n95 = Unbundle By Name(w254) -> ("MPU_Stick_Queues.UI Event Handler"=w253:refnum<queue>)
          n96 = Unbundle By Name(w254) -> ("IMU_configuration_references.Set Accelerometer F.S. Value"=w252:refnum<vi>, "IMU_configuration_references.Set Accelerometer bandwidth"=w251:refnum<vi>, "IMU_configuration_references.Set Gyroscope F.S. Value"=w250:refnum<vi>, "IMU_configuration_references.Set Gyroscope bandwidth"=w249:refnum<vi>, "IMU_configuration_references.Set calibration interval"=w248:refnum<vi>, "IMU_configuration_references.Set calibration point count"=w247:refnum<vi>, "IMU_configuration_references.Set sampling frequency"=w246:refnum<vi>, "IMU_configuration_references.Set all IMU configurations"=w238:refnum<vi>)
          n97 = flat-sequence {
            tunnel: w243 -> [w257]
            tunnel: [w257] -> w242
            tunnel: [w256] -> w239
            frame #0 {
              n98 = local read "IMU Config.Set Parameter Index"() -> (w256:u32)
            }
          }
          n99 = Build Array(w252, w251, w250, w249, w248, w247, w246, w238) -> (w245:refnum<vi>[])
          n100 = for {
            tunnel: w245 -> [w261] mode=indexing
            shift-right: [w260] -> w241
            shift-left: w242 -> [w262]
            tunnel: [w259] -> w237
            tunnel: [w258] -> w233
            i -> [w259]
            stop <- w258 stop-if-true
            n101 = property class="Bool (strict)"(reference=w261, error in=w262) -> (error out=w260:errorcluster, "Value"=w258:bool)  [unwired: 1 out]
          }
          n102 = Increment(x=w237) -> (x+1=w235:i32)
          n103 = Select(t=w235, s=w233, f=0) -> (s? t:f=w236:i32)
          n104 = To Unsigned Long Integer(number=w236) -> (unsigned 32bit integer=w240:u32)
          "IMU Config.Set Parameter Index" <- w240
          n105 = Not Equal?(x=w240, y=w239) -> (x != y?=w255:bool)
          n106 = case shown="True" w255 {
            tunnel: [w263 w269] -> w244
            tunnel: w253 -> [_ w268]
            tunnel: w241 -> [w263 w267]
            tunnel: w240 -> [_ w266]
            tunnel: w239 -> [_ w265]
            frame False {
            }
            frame True {
              w264 = T15[] [enum."IMU_ACCEL_FS", enum."IMU_ACCEL_BW", enum."IMU_GYRO_FS", enum."IMU_GYRO_BW", enum."IMU_CALIB_INTERVAL", enum."IMU_CALIB_POINT_COUNT", enum."IMU_SAMPLING_FREQ"] items=["IMU_ACCEL_FS", "IMU_ACCEL_BW", "IMU_GYRO_FS", "IMU_GYRO_BW", "IMU_CALIB_INTERVAL", "IMU_CALIB_POINT_COUNT", "IMU_SAMPLING_FREQ", "LED1_CONFIG", "LED2_CONFIG", "LED3_CONFIG", "MP_ROLL_FILTER_CONSTANT", "MP_PITCH_FILTER_CONSTANT", "MP_THRESHOLD_X_ACCEL_LOW", "MP_THRESHOLD_X_ACCEL_HIGH", "MP_THRESHOLD_Y_ACCEL_LOW", "MP_THRESHOLD_Y_ACCEL_HIGH", "MP_THRESHOLD_Z_ACCEL_LOW", "MP_THRESHOLD_Z_ACCEL_HIGH", "MP_THRESHOLD_X_GYRO_LOW", "MP_THRESHOLD_X_GYRO_HIGH", "MP_THRESHOLD_Y_GYRO_LOW", "MP_THRESHOLD_Y_GYRO_HIGH", "MP_THRESHOLD_Z_GYRO_LOW", "MP_THRESHOLD_Z_GYRO_HIGH", "MP_THRESHOLD_ROLL_LOW", "MP_THRESHOLD_ROLL_HIGH", "MP_THRESHOLD_PITCH_LOW", "MP_THRESHOLD_PITCH_HIGH", "MP_THRESHOLD_YAW_LOW", "MP_THRESHOLD_YAW_HIGH", "MP_DETECTION_TYPE_X_ACCEL", "MP_DETECTION_TYPE_Y_ACCEL", "MP_DETECTION_TYPE_Z_ACCEL", "MP_DETECTION_TYPE_X_GYRO", "MP_DETECTION_TYPE_Y_GYRO", "MP_DETECTION_TYPE_Z_GYRO", "MP_DETECTION_TYPE_ROLL", "MP_DETECTION_TYPE_PITCH", "MP_DETECTION_TYPE_YAW"]
              n107 = property on="IMU Config.Set Parameter Index" class="DigNum (strict)"(error in=w267, "Val(Sgnl)"=w266) -> (error out=w270:errorcluster)  [unwired: 1 in, 1 out]
              n108 = case shown="8" w265 {
                selector: w265 -> [w273 _ _]
                tunnel: w270 -> [w280 w284 w292]
                tunnel: [w279 w283 w292] -> w269
                tunnel: w268 -> [w278 w282 _]
                tunnel: w264 -> [w274 w281 _]
                frame 1..7 {
                  n109 = Decrement(x=w273) -> (x-1=w271:u32)
                  n110 = Index Array(array=w274, index=w271) -> (element=w272:T15)
                  n111 = To Variant(anything=w272) -> (Variant=w275:variant)
                  n112 = Bundle By Name(cluster=T11 {"Data"=variant, "Command"=enum."UI_Event_Set_Config_RQST"} ("element"), "Data"=w275) -> (w276:T11)
                  n113 = Enqueue Element(queue=w278, element=w276, error in (no error)=w280) -> (error out=w279:errorcluster)  [unwired: 1 in, 2 out]
                }
                frame 8 {
                  n114 = for {
                    tunnel: w282 -> [w289]
                    shift-right: [w290] -> w283
                    shift-left: w284 -> [w291]
                    tunnel: w281 -> [w285] mode=indexing
                    n115 = To Variant(anything=w285) -> (Variant=w286:variant)
                    n116 = Bundle By Name(cluster=T11 {"Data"=variant, "Command"=enum."UI_Event_Set_Config_RQST"} ("element"), "Data"=w286) -> (w287:T11)
                    n117 = Enqueue Element(queue=w289, element=w287, error in (no error)=w291) -> (error out=w290:errorcluster)  [unwired: 1 in, 2 out]
                  }
                }
                frame Default {
                }
              }
            }
          }
        }
        frame "LED_CONFIG_GET" {
          n118 = Unbundle By Name(w297) -> ("MPU_Stick_Queues.UI Event Handler"=w310:refnum<queue>)
          n119 = Unbundle By Name(w297) -> ("LED_Configuration_References.Get LED1 configuration"=w296:refnum<vi>, "LED_Configuration_References.Get LED2 configuration"=w295:refnum<vi>, "LED_Configuration_References.Get LED3 configuration"=w294:refnum<vi>, "LED_Configuration_References.Get all LED configurations"=w293:refnum<vi>)
          n120 = flat-sequence {
            tunnel: w307 -> [w313]
            tunnel: [w313] -> w306
            tunnel: [w312] -> w303
            frame #0 {
              n121 = local read "LED Config.Get Parameter Index"() -> (w312:u32)
            }
          }
          n122 = Build Array(w296, w295, w294, w293) -> (w309:refnum<vi>[])
          n123 = for {
            tunnel: w309 -> [w314] mode=indexing
            shift-right: [w317] -> w305
            shift-left: w306 -> [w318]
            tunnel: [w316] -> w302
            tunnel: [w315] -> w298
            i -> [w316]
            stop <- w315 stop-if-true
            n124 = property class="Bool (strict)"(reference=w314, error in=w318) -> (error out=w317:errorcluster, "Value"=w315:bool)  [unwired: 1 out]
          }
          n125 = Increment(x=w302) -> (x+1=w300:i32)
          n126 = Select(t=w300, s=w298, f=0) -> (s? t:f=w301:i32)
          n127 = To Unsigned Long Integer(number=w301) -> (unsigned 32bit integer=w304:u32)
          "LED Config.Get Parameter Index" <- w304
          n128 = Not Equal?(x=w304, y=w303) -> (x != y?=w311:bool)
          n129 = case shown="True" w311 {
            tunnel: [w319 w325] -> w308
            tunnel: w310 -> [_ w324]
            tunnel: w305 -> [w319 w323]
            tunnel: w304 -> [_ w322]
            tunnel: w303 -> [_ w321]
            frame False {
            }
            frame True {
              w320 = T15[] [enum."LED1_CONFIG", enum."LED2_CONFIG", enum."LED3_CONFIG"] items=["IMU_ACCEL_FS", "IMU_ACCEL_BW", "IMU_GYRO_FS", "IMU_GYRO_BW", "IMU_CALIB_INTERVAL", "IMU_CALIB_POINT_COUNT", "IMU_SAMPLING_FREQ", "LED1_CONFIG", "LED2_CONFIG", "LED3_CONFIG", "MP_ROLL_FILTER_CONSTANT", "MP_PITCH_FILTER_CONSTANT", "MP_THRESHOLD_X_ACCEL_LOW", "MP_THRESHOLD_X_ACCEL_HIGH", "MP_THRESHOLD_Y_ACCEL_LOW", "MP_THRESHOLD_Y_ACCEL_HIGH", "MP_THRESHOLD_Z_ACCEL_LOW", "MP_THRESHOLD_Z_ACCEL_HIGH", "MP_THRESHOLD_X_GYRO_LOW", "MP_THRESHOLD_X_GYRO_HIGH", "MP_THRESHOLD_Y_GYRO_LOW", "MP_THRESHOLD_Y_GYRO_HIGH", "MP_THRESHOLD_Z_GYRO_LOW", "MP_THRESHOLD_Z_GYRO_HIGH", "MP_THRESHOLD_ROLL_LOW", "MP_THRESHOLD_ROLL_HIGH", "MP_THRESHOLD_PITCH_LOW", "MP_THRESHOLD_PITCH_HIGH", "MP_THRESHOLD_YAW_LOW", "MP_THRESHOLD_YAW_HIGH", "MP_DETECTION_TYPE_X_ACCEL", "MP_DETECTION_TYPE_Y_ACCEL", "MP_DETECTION_TYPE_Z_ACCEL", "MP_DETECTION_TYPE_X_GYRO", "MP_DETECTION_TYPE_Y_GYRO", "MP_DETECTION_TYPE_Z_GYRO", "MP_DETECTION_TYPE_ROLL", "MP_DETECTION_TYPE_PITCH", "MP_DETECTION_TYPE_YAW"]
              n130 = property on="LED Config.Get Parameter Index" class="DigNum (strict)"(error in=w323, "Val(Sgnl)"=w322) -> (error out=w326:errorcluster)  [unwired: 1 in, 1 out]
              n131 = case shown="4" w321 {
                selector: w321 -> [w329 _ _]
                tunnel: w326 -> [w336 w340 w348]
                tunnel: [w335 w339 w348] -> w325
                tunnel: w324 -> [w334 w338 _]
                tunnel: w320 -> [w330 w337 _]
                frame 1..3 {
                  n132 = Decrement(x=w329) -> (x-1=w327:u32)
                  n133 = Index Array(array=w330, index=w327) -> (element=w328:T15)
                  n134 = To Variant(anything=w328) -> (Variant=w331:variant)
                  n135 = Bundle By Name(cluster=T11 {"Data"=variant, "Command"=enum."UI_Event_Get_Config_RQST"} ("element"), "Data"=w331) -> (w332:T11)
                  n136 = Enqueue Element(queue=w334, element=w332, error in (no error)=w336) -> (error out=w335:errorcluster)  [unwired: 1 in, 2 out]
                }
                frame 4 {
                  n137 = for {
                    tunnel: w338 -> [w345]
                    shift-right: [w346] -> w339
                    shift-left: w340 -> [w347]
                    tunnel: w337 -> [w341] mode=indexing
                    n138 = To Variant(anything=w341) -> (Variant=w342:variant)
                    n139 = Bundle By Name(cluster=T11 {"Data"=variant, "Command"=enum."UI_Event_Get_Config_RQST"} ("element"), "Data"=w342) -> (w343:T11)
                    n140 = Enqueue Element(queue=w345, element=w343, error in (no error)=w347) -> (error out=w346:errorcluster)  [unwired: 1 in, 2 out]
                  }
                }
                frame Default {
                }
              }
            }
          }
        }
        frame "LED_CONFIG_SET" {
          n141 = Unbundle By Name(w353) -> ("MPU_Stick_Queues.UI Event Handler"=w366:refnum<queue>)
          n142 = Unbundle By Name(w353) -> ("LED_Configuration_References.Set LED1 configuration"=w352:refnum<vi>, "LED_Configuration_References.Set LED2 configuration"=w351:refnum<vi>, "LED_Configuration_References.Set LED3 configuration"=w350:refnum<vi>, "LED_Configuration_References.Set all LED configurations"=w349:refnum<vi>)
          n143 = flat-sequence {
            tunnel: w363 -> [w369]
            tunnel: [w369] -> w362
            tunnel: [w368] -> w359
            frame #0 {
              n144 = local read "LED Config.Set Parameter Index"() -> (w368:u32)
            }
          }
          n145 = Build Array(w352, w351, w350, w349) -> (w365:refnum<vi>[])
          n146 = for {
            tunnel: w365 -> [w370] mode=indexing
            shift-right: [w373] -> w361
            shift-left: w362 -> [w374]
            tunnel: [w372] -> w358
            tunnel: [w371] -> w354
            i -> [w372]
            stop <- w371 stop-if-true
            n147 = property class="Bool (strict)"(reference=w370, error in=w374) -> (error out=w373:errorcluster, "Value"=w371:bool)  [unwired: 1 out]
          }
          n148 = Increment(x=w358) -> (x+1=w356:i32)
          n149 = Select(t=w356, s=w354, f=0) -> (s? t:f=w357:i32)
          n150 = To Unsigned Long Integer(number=w357) -> (unsigned 32bit integer=w360:u32)
          "LED Config.Set Parameter Index" <- w360
          n151 = Not Equal?(x=w360, y=w359) -> (x != y?=w367:bool)
          n152 = case shown="True" w367 {
            tunnel: [w375 w381] -> w364
            tunnel: w366 -> [_ w380]
            tunnel: w361 -> [w375 w379]
            tunnel: w360 -> [_ w378]
            tunnel: w359 -> [_ w377]
            frame False {
            }
            frame True {
              w376 = T15[] [enum."LED1_CONFIG", enum."LED2_CONFIG", enum."LED3_CONFIG"] items=["IMU_ACCEL_FS", "IMU_ACCEL_BW", "IMU_GYRO_FS", "IMU_GYRO_BW", "IMU_CALIB_INTERVAL", "IMU_CALIB_POINT_COUNT", "IMU_SAMPLING_FREQ", "LED1_CONFIG", "LED2_CONFIG", "LED3_CONFIG", "MP_ROLL_FILTER_CONSTANT", "MP_PITCH_FILTER_CONSTANT", "MP_THRESHOLD_X_ACCEL_LOW", "MP_THRESHOLD_X_ACCEL_HIGH", "MP_THRESHOLD_Y_ACCEL_LOW", "MP_THRESHOLD_Y_ACCEL_HIGH", "MP_THRESHOLD_Z_ACCEL_LOW", "MP_THRESHOLD_Z_ACCEL_HIGH", "MP_THRESHOLD_X_GYRO_LOW", "MP_THRESHOLD_X_GYRO_HIGH", "MP_THRESHOLD_Y_GYRO_LOW", "MP_THRESHOLD_Y_GYRO_HIGH", "MP_THRESHOLD_Z_GYRO_LOW", "MP_THRESHOLD_Z_GYRO_HIGH", "MP_THRESHOLD_ROLL_LOW", "MP_THRESHOLD_ROLL_HIGH", "MP_THRESHOLD_PITCH_LOW", "MP_THRESHOLD_PITCH_HIGH", "MP_THRESHOLD_YAW_LOW", "MP_THRESHOLD_YAW_HIGH", "MP_DETECTION_TYPE_X_ACCEL", "MP_DETECTION_TYPE_Y_ACCEL", "MP_DETECTION_TYPE_Z_ACCEL", "MP_DETECTION_TYPE_X_GYRO", "MP_DETECTION_TYPE_Y_GYRO", "MP_DETECTION_TYPE_Z_GYRO", "MP_DETECTION_TYPE_ROLL", "MP_DETECTION_TYPE_PITCH", "MP_DETECTION_TYPE_YAW"]
              n153 = property on="LED Config.Set Parameter Index" class="DigNum (strict)"(error in=w379, "Val(Sgnl)"=w378) -> (error out=w382:errorcluster)  [unwired: 1 in, 1 out]
              n154 = case shown="4" w377 {
                selector: w377 -> [w385 _ _]
                tunnel: w382 -> [w392 w396 w404]
                tunnel: [w391 w395 w404] -> w381
                tunnel: w380 -> [w390 w394 _]
                tunnel: w376 -> [w386 w393 _]
                frame 1..3 {
                  n155 = Decrement(x=w385) -> (x-1=w383:u32)
                  n156 = Index Array(array=w386, index=w383) -> (element=w384:T15)
                  n157 = To Variant(anything=w384) -> (Variant=w387:variant)
                  n158 = Bundle By Name(cluster=T11 {"Data"=variant, "Command"=enum."UI_Event_Set_Config_RQST"} ("element"), "Data"=w387) -> (w388:T11)
                  n159 = Enqueue Element(queue=w390, element=w388, error in (no error)=w392) -> (error out=w391:errorcluster)  [unwired: 1 in, 2 out]
                }
                frame 4 {
                  n160 = for {
                    tunnel: w394 -> [w401]
                    shift-right: [w402] -> w395
                    shift-left: w396 -> [w403]
                    tunnel: w393 -> [w397] mode=indexing
                    n161 = To Variant(anything=w397) -> (Variant=w398:variant)
                    n162 = Bundle By Name(cluster=T11 {"Data"=variant, "Command"=enum."UI_Event_Set_Config_RQST"} ("element"), "Data"=w398) -> (w399:T11)
                    n163 = Enqueue Element(queue=w401, element=w399, error in (no error)=w403) -> (error out=w402:errorcluster)  [unwired: 1 in, 2 out]
                  }
                }
                frame Default {
                }
              }
            }
          }
        }
        frame "FILTER_CONSTANTS_GET" {
          n164 = Unbundle By Name(w407) -> ("MPU_Stick_Queues.UI Event Handler"=w420:refnum<queue>)
          n165 = Unbundle By Name(w407) -> ("MP_Comp_Filter_Constants_References.Get roll filter constant"=w406:refnum<vi>, "MP_Comp_Filter_Constants_References.Get pitch filter constant"=w405:refnum<vi>)
          n166 = flat-sequence {
            tunnel: w417 -> [w423]
            tunnel: [w423] -> w416
            tunnel: [w422] -> w413
            frame #0 {
              n167 = local read "Filter constants Config.Get Parameter Index"() -> (w422:u32)
            }
          }
          n168 = Build Array(w406, w405) -> (w419:refnum<vi>[])
          n169 = for {
            tunnel: w419 -> [w424] mode=indexing
            shift-right: [w427] -> w415
            shift-left: w416 -> [w428]
            tunnel: [w426] -> w412
            tunnel: [w425] -> w408
            i -> [w426]
            stop <- w425 stop-if-true
            n170 = property class="Bool (strict)"(reference=w424, error in=w428) -> (error out=w427:errorcluster, "Value"=w425:bool)  [unwired: 1 out]
          }
          n171 = Increment(x=w412) -> (x+1=w410:i32)
          n172 = Select(t=w410, s=w408, f=0) -> (s? t:f=w411:i32)
          n173 = To Unsigned Long Integer(number=w411) -> (unsigned 32bit integer=w414:u32)
          "Filter constants Config.Get Parameter Index" <- w414
          n174 = Not Equal?(x=w414, y=w413) -> (x != y?=w421:bool)
          n175 = case shown="True" w421 {
            tunnel: [w429 w435] -> w418
            tunnel: w420 -> [_ w434]
            tunnel: w415 -> [w429 w433]
            tunnel: w414 -> [_ w432]
            tunnel: w413 -> [_ w431]
            frame False {
            }
            frame True {
              w430 = T15[] [enum."MP_ROLL_FILTER_CONSTANT", enum."MP_PITCH_FILTER_CONSTANT"] items=["IMU_ACCEL_FS", "IMU_ACCEL_BW", "IMU_GYRO_FS", "IMU_GYRO_BW", "IMU_CALIB_INTERVAL", "IMU_CALIB_POINT_COUNT", "IMU_SAMPLING_FREQ", "LED1_CONFIG", "LED2_CONFIG", "LED3_CONFIG", "MP_ROLL_FILTER_CONSTANT", "MP_PITCH_FILTER_CONSTANT", "MP_THRESHOLD_X_ACCEL_LOW", "MP_THRESHOLD_X_ACCEL_HIGH", "MP_THRESHOLD_Y_ACCEL_LOW", "MP_THRESHOLD_Y_ACCEL_HIGH", "MP_THRESHOLD_Z_ACCEL_LOW", "MP_THRESHOLD_Z_ACCEL_HIGH", "MP_THRESHOLD_X_GYRO_LOW", "MP_THRESHOLD_X_GYRO_HIGH", "MP_THRESHOLD_Y_GYRO_LOW", "MP_THRESHOLD_Y_GYRO_HIGH", "MP_THRESHOLD_Z_GYRO_LOW", "MP_THRESHOLD_Z_GYRO_HIGH", "MP_THRESHOLD_ROLL_LOW", "MP_THRESHOLD_ROLL_HIGH", "MP_THRESHOLD_PITCH_LOW", "MP_THRESHOLD_PITCH_HIGH", "MP_THRESHOLD_YAW_LOW", "MP_THRESHOLD_YAW_HIGH", "MP_DETECTION_TYPE_X_ACCEL", "MP_DETECTION_TYPE_Y_ACCEL", "MP_DETECTION_TYPE_Z_ACCEL", "MP_DETECTION_TYPE_X_GYRO", "MP_DETECTION_TYPE_Y_GYRO", "MP_DETECTION_TYPE_Z_GYRO", "MP_DETECTION_TYPE_ROLL", "MP_DETECTION_TYPE_PITCH", "MP_DETECTION_TYPE_YAW"]
              n176 = property on="Filter constants Config.Get Parameter Index" class="DigNum (strict)"(error in=w433, "Val(Sgnl)"=w432) -> (error out=w436:errorcluster)  [unwired: 1 in, 1 out]
              n177 = case shown="4" w431 {
                selector: w431 -> [w439 _ _]
                tunnel: w436 -> [w446 w450 w458]
                tunnel: [w445 w449 w458] -> w435
                tunnel: w434 -> [w444 w448 _]
                tunnel: w430 -> [w440 w447 _]
                frame 1..3 {
                  n178 = Decrement(x=w439) -> (x-1=w437:u32)
                  n179 = Index Array(array=w440, index=w437) -> (element=w438:T15)
                  n180 = To Variant(anything=w438) -> (Variant=w441:variant)
                  n181 = Bundle By Name(cluster=T11 {"Data"=variant, "Command"=enum."UI_Event_Get_Config_RQST"} ("element"), "Data"=w441) -> (w442:T11)
                  n182 = Enqueue Element(queue=w444, element=w442, error in (no error)=w446) -> (error out=w445:errorcluster)  [unwired: 1 in, 2 out]
                }
                frame 4 {
                  n183 = for {
                    tunnel: w448 -> [w455]
                    shift-right: [w456] -> w449
                    shift-left: w450 -> [w457]
                    tunnel: w447 -> [w451] mode=indexing
                    n184 = To Variant(anything=w451) -> (Variant=w452:variant)
                    n185 = Bundle By Name(cluster=T11 {"Data"=variant, "Command"=enum."UI_Event_Get_Config_RQST"} ("element"), "Data"=w452) -> (w453:T11)
                    n186 = Enqueue Element(queue=w455, element=w453, error in (no error)=w457) -> (error out=w456:errorcluster)  [unwired: 1 in, 2 out]
                  }
                }
                frame Default {
                }
              }
            }
          }
        }
        frame "FILTER_CONSTANTS_SET" {
          n187 = Unbundle By Name(w461) -> ("MPU_Stick_Queues.UI Event Handler"=w474:refnum<queue>)
          n188 = Unbundle By Name(w461) -> ("MP_Comp_Filter_Constants_References.Set roll filter constant"=w460:refnum<vi>, "MP_Comp_Filter_Constants_References.Set pitch filter constant"=w459:refnum<vi>)
          n189 = flat-sequence {
            tunnel: w471 -> [w477]
            tunnel: [w477] -> w470
            tunnel: [w476] -> w467
            frame #0 {
              n190 = local read "Filter constants Config.Set Parameter Index"() -> (w476:u32)
            }
          }
          n191 = Build Array(w460, w459) -> (w473:refnum<vi>[])
          n192 = for {
            tunnel: w473 -> [w478] mode=indexing
            shift-right: [w481] -> w469
            shift-left: w470 -> [w482]
            tunnel: [w480] -> w466
            tunnel: [w479] -> w462
            i -> [w480]
            stop <- w479 stop-if-true
            n193 = property class="Bool (strict)"(reference=w478, error in=w482) -> (error out=w481:errorcluster, "Value"=w479:bool)  [unwired: 1 out]
          }
          n194 = Increment(x=w466) -> (x+1=w464:i32)
          n195 = Select(t=w464, s=w462, f=0) -> (s? t:f=w465:i32)
          n196 = To Unsigned Long Integer(number=w465) -> (unsigned 32bit integer=w468:u32)
          "Filter constants Config.Set Parameter Index" <- w468
          n197 = Not Equal?(x=w468, y=w467) -> (x != y?=w475:bool)
          n198 = case shown="True" w475 {
            tunnel: [w483 w489] -> w472
            tunnel: w474 -> [_ w488]
            tunnel: w469 -> [w483 w487]
            tunnel: w468 -> [_ w486]
            tunnel: w467 -> [_ w485]
            frame False {
            }
            frame True {
              w484 = T15[] [enum."MP_ROLL_FILTER_CONSTANT", enum."MP_PITCH_FILTER_CONSTANT"] items=["IMU_ACCEL_FS", "IMU_ACCEL_BW", "IMU_GYRO_FS", "IMU_GYRO_BW", "IMU_CALIB_INTERVAL", "IMU_CALIB_POINT_COUNT", "IMU_SAMPLING_FREQ", "LED1_CONFIG", "LED2_CONFIG", "LED3_CONFIG", "MP_ROLL_FILTER_CONSTANT", "MP_PITCH_FILTER_CONSTANT", "MP_THRESHOLD_X_ACCEL_LOW", "MP_THRESHOLD_X_ACCEL_HIGH", "MP_THRESHOLD_Y_ACCEL_LOW", "MP_THRESHOLD_Y_ACCEL_HIGH", "MP_THRESHOLD_Z_ACCEL_LOW", "MP_THRESHOLD_Z_ACCEL_HIGH", "MP_THRESHOLD_X_GYRO_LOW", "MP_THRESHOLD_X_GYRO_HIGH", "MP_THRESHOLD_Y_GYRO_LOW", "MP_THRESHOLD_Y_GYRO_HIGH", "MP_THRESHOLD_Z_GYRO_LOW", "MP_THRESHOLD_Z_GYRO_HIGH", "MP_THRESHOLD_ROLL_LOW", "MP_THRESHOLD_ROLL_HIGH", "MP_THRESHOLD_PITCH_LOW", "MP_THRESHOLD_PITCH_HIGH", "MP_THRESHOLD_YAW_LOW", "MP_THRESHOLD_YAW_HIGH", "MP_DETECTION_TYPE_X_ACCEL", "MP_DETECTION_TYPE_Y_ACCEL", "MP_DETECTION_TYPE_Z_ACCEL", "MP_DETECTION_TYPE_X_GYRO", "MP_DETECTION_TYPE_Y_GYRO", "MP_DETECTION_TYPE_Z_GYRO", "MP_DETECTION_TYPE_ROLL", "MP_DETECTION_TYPE_PITCH", "MP_DETECTION_TYPE_YAW"]
              n199 = property on="Filter constants Config.Set Parameter Index" class="DigNum (strict)"(error in=w487, "Val(Sgnl)"=w486) -> (error out=w490:errorcluster)  [unwired: 1 in, 1 out]
              n200 = case shown="4" w485 {
                selector: w485 -> [w493 _ _]
                tunnel: w490 -> [w500 w504 w512]
                tunnel: [w499 w503 w512] -> w489
                tunnel: w488 -> [w498 w502 _]
                tunnel: w484 -> [w494 w501 _]
                frame 1..3 {
                  n201 = Decrement(x=w493) -> (x-1=w491:u32)
                  n202 = Index Array(array=w494, index=w491) -> (element=w492:T15)
                  n203 = To Variant(anything=w492) -> (Variant=w495:variant)
                  n204 = Bundle By Name(cluster=T11 {"Data"=variant, "Command"=enum."UI_Event_Set_Config_RQST"} ("element"), "Data"=w495) -> (w496:T11)
                  n205 = Enqueue Element(queue=w498, element=w496, error in (no error)=w500) -> (error out=w499:errorcluster)  [unwired: 1 in, 2 out]
                }
                frame 4 {
                  n206 = for {
                    tunnel: w502 -> [w509]
                    shift-right: [w510] -> w503
                    shift-left: w504 -> [w511]
                    tunnel: w501 -> [w505] mode=indexing
                    n207 = To Variant(anything=w505) -> (Variant=w506:variant)
                    n208 = Bundle By Name(cluster=T11 {"Data"=variant, "Command"=enum."UI_Event_Set_Config_RQST"} ("element"), "Data"=w506) -> (w507:T11)
                    n209 = Enqueue Element(queue=w509, element=w507, error in (no error)=w511) -> (error out=w510:errorcluster)  [unwired: 1 in, 2 out]
                  }
                }
                frame Default {
                }
              }
            }
          }
        }
        frame "MD_THRESHOLDS_GET" {
          n210 = Unbundle By Name(w532) -> ("MD_Threshold_References.Get yaw threshold (upper)"=w531:refnum<vi>, "MD_Threshold_References.Get yaw threshold (lower)"=w530:refnum<vi>, "MD_Threshold_References.Get pitch threshold (upper)"=w529:refnum<vi>, "MD_Threshold_References.Get pitch threshold (lower)"=w528:refnum<vi>, "MD_Threshold_References.Get roll threshold (upper)"=w527:refnum<vi>, "MD_Threshold_References.Get roll threshold (lower)"=w526:refnum<vi>, "MD_Threshold_References.Get Z gyro threshold (upper)"=w525:refnum<vi>, "MD_Threshold_References.Get Z gyro threshold (lower)"=w524:refnum<vi>, "MD_Threshold_References.Get Y gyro threshold (upper)"=w523:refnum<vi>, "MD_Threshold_References.Get Y gyro threshold (lower)"=w522:refnum<vi>, "MD_Threshold_References.Get X gyro threshold (upper)"=w521:refnum<vi>, "MD_Threshold_References.Get X gyro threshold (lower)"=w520:refnum<vi>, "MD_Threshold_References.Get Z accel threshold (upper)"=w519:refnum<vi>, "MD_Threshold_References.Get Z accel threshold (lower)"=w518:refnum<vi>, "MD_Threshold_References.Get Y accel threshold (upper)"=w517:refnum<vi>, "MD_Threshold_References.Get Y accel threshold (lower)"=w516:refnum<vi>, "MD_Threshold_References.Get X accel threshold (upper)"=w515:refnum<vi>, "MD_Threshold_References.Get X accel threshold (lower)"=w514:refnum<vi>, "MD_Threshold_References.Get all Motion detection threshold configurations"=w513:refnum<vi>)
          n211 = Unbundle By Name(w532) -> ("MPU_Stick_Queues.UI Event Handler"=w545:refnum<queue>)
          n212 = flat-sequence {
            tunnel: w542 -> [w548]
            tunnel: [w548] -> w541
            tunnel: [w547] -> w538
            frame #0 {
              n213 = local read "MD Thresholds Config.Set Parameter Index"() -> (w547:u32)
            }
          }
          n214 = Build Array(w531, w530, w529, w528, w527, w526, w525, w524, w523, w522, w521, w520, w519, w518, w517, w516, w515, w514, w513) -> (w544:refnum<vi>[])
          n215 = for {
            tunnel: w544 -> [w549] mode=indexing
            shift-right: [w552] -> w540
            shift-left: w541 -> [w553]
            tunnel: [w551] -> w537
            tunnel: [w550] -> w533
            i -> [w551]
            stop <- w550 stop-if-true
            n216 = property class="Bool (strict)"(reference=w549, error in=w553) -> (error out=w552:errorcluster, "Value"=w550:bool)  [unwired: 1 out]
          }
          n217 = Increment(x=w537) -> (x+1=w535:i32)
          n218 = Select(t=w535, s=w533, f=0) -> (s? t:f=w536:i32)
          n219 = To Unsigned Long Integer(number=w536) -> (unsigned 32bit integer=w539:u32)
          "MD Thresholds Config.Set Parameter Index" <- w539
          n220 = Not Equal?(x=w539, y=w538) -> (x != y?=w546:bool)
          n221 = case shown="True" w546 {
            tunnel: [w554 w560] -> w543
            tunnel: w545 -> [_ w559]
            tunnel: w540 -> [w554 w558]
            tunnel: w539 -> [_ w557]
            tunnel: w538 -> [_ w556]
            frame False {
            }
            frame True {
              w555 = T15[] [enum."MP_THRESHOLD_YAW_HIGH", enum."MP_THRESHOLD_YAW_LOW", enum."MP_THRESHOLD_PITCH_HIGH", enum."MP_THRESHOLD_PITCH_LOW", enum."MP_THRESHOLD_ROLL_HIGH", enum."MP_THRESHOLD_ROLL_LOW", enum."MP_THRESHOLD_Z_GYRO_HIGH", enum."MP_THRESHOLD_Z_GYRO_LOW", enum."MP_THRESHOLD_Y_GYRO_HIGH", enum."MP_THRESHOLD_Y_GYRO_LOW", enum."MP_THRESHOLD_X_GYRO_HIGH", enum."MP_THRESHOLD_X_GYRO_LOW", enum."MP_THRESHOLD_Z_ACCEL_HIGH", enum."MP_THRESHOLD_Z_ACCEL_LOW", enum."MP_THRESHOLD_Y_ACCEL_HIGH", enum."MP_THRESHOLD_Y_ACCEL_LOW", enum."MP_THRESHOLD_X_ACCEL_HIGH", enum."MP_THRESHOLD_X_ACCEL_LOW"] items=["IMU_ACCEL_FS", "IMU_ACCEL_BW", "IMU_GYRO_FS", "IMU_GYRO_BW", "IMU_CALIB_INTERVAL", "IMU_CALIB_POINT_COUNT", "IMU_SAMPLING_FREQ", "LED1_CONFIG", "LED2_CONFIG", "LED3_CONFIG", "MP_ROLL_FILTER_CONSTANT", "MP_PITCH_FILTER_CONSTANT", "MP_THRESHOLD_X_ACCEL_LOW", "MP_THRESHOLD_X_ACCEL_HIGH", "MP_THRESHOLD_Y_ACCEL_LOW", "MP_THRESHOLD_Y_ACCEL_HIGH", "MP_THRESHOLD_Z_ACCEL_LOW", "MP_THRESHOLD_Z_ACCEL_HIGH", "MP_THRESHOLD_X_GYRO_LOW", "MP_THRESHOLD_X_GYRO_HIGH", "MP_THRESHOLD_Y_GYRO_LOW", "MP_THRESHOLD_Y_GYRO_HIGH", "MP_THRESHOLD_Z_GYRO_LOW", "MP_THRESHOLD_Z_GYRO_HIGH", "MP_THRESHOLD_ROLL_LOW", "MP_THRESHOLD_ROLL_HIGH", "MP_THRESHOLD_PITCH_LOW", "MP_THRESHOLD_PITCH_HIGH", "MP_THRESHOLD_YAW_LOW", "MP_THRESHOLD_YAW_HIGH", "MP_DETECTION_TYPE_X_ACCEL", "MP_DETECTION_TYPE_Y_ACCEL", "MP_DETECTION_TYPE_Z_ACCEL", "MP_DETECTION_TYPE_X_GYRO", "MP_DETECTION_TYPE_Y_GYRO", "MP_DETECTION_TYPE_Z_GYRO", "MP_DETECTION_TYPE_ROLL", "MP_DETECTION_TYPE_PITCH", "MP_DETECTION_TYPE_YAW"]
              n222 = property on="MD Thresholds Config.Set Parameter Index" class="DigNum (strict)"(error in=w558, "Val(Sgnl)"=w557) -> (error out=w561:errorcluster)  [unwired: 1 in, 1 out]
              n223 = case shown="19" w556 {
                selector: w556 -> [w564 _ _]
                tunnel: w561 -> [w571 w575 w583]
                tunnel: [w570 w574 w583] -> w560
                tunnel: w559 -> [w569 w573 _]
                tunnel: w555 -> [w565 w572 _]
                frame 1..18 {
                  n224 = Decrement(x=w564) -> (x-1=w562:u32)
                  n225 = Index Array(array=w565, index=w562) -> (element=w563:T15)
                  n226 = To Variant(anything=w563) -> (Variant=w566:variant)
                  n227 = Bundle By Name(cluster=T11 {"Data"=variant, "Command"=enum."UI_Event_Get_Config_RQST"} ("element"), "Data"=w566) -> (w567:T11)
                  n228 = Enqueue Element(queue=w569, element=w567, error in (no error)=w571) -> (error out=w570:errorcluster)  [unwired: 1 in, 2 out]
                }
                frame 19 {
                  n229 = for {
                    tunnel: w573 -> [w580]
                    shift-right: [w581] -> w574
                    shift-left: w575 -> [w582]
                    tunnel: w572 -> [w576] mode=indexing
                    n230 = To Variant(anything=w576) -> (Variant=w577:variant)
                    n231 = Bundle By Name(cluster=T11 {"Data"=variant, "Command"=enum."UI_Event_Get_Config_RQST"} ("element"), "Data"=w577) -> (w578:T11)
                    n232 = Enqueue Element(queue=w580, element=w578, error in (no error)=w582) -> (error out=w581:errorcluster)  [unwired: 1 in, 2 out]
                  }
                }
                frame Default {
                }
              }
            }
          }
        }
        frame "MD_THRESHOLDS_SET" {
          n233 = Unbundle By Name(w603) -> ("MD_Threshold_References.Set yaw threshold (upper)"=w602:refnum<vi>, "MD_Threshold_References.Set yaw threshold (lower)"=w601:refnum<vi>, "MD_Threshold_References.Set pitch threshold (upper)"=w600:refnum<vi>, "MD_Threshold_References.Set pitch threshold (lower)"=w599:refnum<vi>, "MD_Threshold_References.Set roll threshold (upper)"=w598:refnum<vi>, "MD_Threshold_References.Set roll threshold (lower)"=w597:refnum<vi>, "MD_Threshold_References.Set Z gyro threshold (upper)"=w596:refnum<vi>, "MD_Threshold_References.Set Z gyro threshold (lower)"=w595:refnum<vi>, "MD_Threshold_References.Set Y gyro threshold (upper)"=w594:refnum<vi>, "MD_Threshold_References.Set Y gyro threshold (lower)"=w593:refnum<vi>, "MD_Threshold_References.Set X gyro threshold (upper)"=w592:refnum<vi>, "MD_Threshold_References.Set X gyro threshold (lower)"=w591:refnum<vi>, "MD_Threshold_References.Set Z accel threshold (upper)"=w590:refnum<vi>, "MD_Threshold_References.Set Z accel threshold (lower)"=w589:refnum<vi>, "MD_Threshold_References.Set Y accel threshold (upper)"=w588:refnum<vi>, "MD_Threshold_References.Set Y accel threshold (lower)"=w587:refnum<vi>, "MD_Threshold_References.Set X accel threshold (upper)"=w586:refnum<vi>, "MD_Threshold_References.Set X accel threshold (lower)"=w585:refnum<vi>, "MD_Threshold_References.Set all Motion detection threshold configurations"=w584:refnum<vi>)
          n234 = Unbundle By Name(w603) -> ("MPU_Stick_Queues.UI Event Handler"=w616:refnum<queue>)
          n235 = flat-sequence {
            tunnel: w613 -> [w619]
            tunnel: [w619] -> w612
            tunnel: [w618] -> w609
            frame #0 {
              n236 = local read "MD Thresholds Config.Get Parameter Index"() -> (w618:u32)
            }
          }
          n237 = Build Array(w602, w601, w600, w599, w598, w597, w596, w595, w594, w593, w592, w591, w590, w589, w588, w587, w586, w585, w584) -> (w615:refnum<vi>[])
          n238 = for {
            tunnel: w615 -> [w620] mode=indexing
            shift-right: [w623] -> w611
            shift-left: w612 -> [w624]
            tunnel: [w622] -> w608
            tunnel: [w621] -> w604
            i -> [w622]
            stop <- w621 stop-if-true
            n239 = property class="Bool (strict)"(reference=w620, error in=w624) -> (error out=w623:errorcluster, "Value"=w621:bool)  [unwired: 1 out]
          }
          n240 = Increment(x=w608) -> (x+1=w606:i32)
          n241 = Select(t=w606, s=w604, f=0) -> (s? t:f=w607:i32)
          n242 = To Unsigned Long Integer(number=w607) -> (unsigned 32bit integer=w610:u32)
          "MD Thresholds Config.Get Parameter Index" <- w610
          n243 = Not Equal?(x=w610, y=w609) -> (x != y?=w617:bool)
          n244 = case shown="True" w617 {
            tunnel: [w625 w631] -> w614
            tunnel: w616 -> [_ w630]
            tunnel: w611 -> [w625 w629]
            tunnel: w610 -> [_ w628]
            tunnel: w609 -> [_ w627]
            frame False {
            }
            frame True {
              w626 = T15[] [enum."MP_THRESHOLD_YAW_HIGH", enum."MP_THRESHOLD_YAW_LOW", enum."MP_THRESHOLD_PITCH_HIGH", enum."MP_THRESHOLD_PITCH_LOW", enum."MP_THRESHOLD_ROLL_HIGH", enum."MP_THRESHOLD_ROLL_LOW", enum."MP_THRESHOLD_Z_GYRO_HIGH", enum."MP_THRESHOLD_Z_GYRO_LOW", enum."MP_THRESHOLD_Y_GYRO_HIGH", enum."MP_THRESHOLD_Y_GYRO_LOW", enum."MP_THRESHOLD_X_GYRO_HIGH", enum."MP_THRESHOLD_X_GYRO_LOW", enum."MP_THRESHOLD_Z_ACCEL_HIGH", enum."MP_THRESHOLD_Z_ACCEL_LOW", enum."MP_THRESHOLD_Y_ACCEL_HIGH", enum."MP_THRESHOLD_Y_ACCEL_LOW", enum."MP_THRESHOLD_X_ACCEL_HIGH", enum."MP_THRESHOLD_X_ACCEL_LOW"] items=["IMU_ACCEL_FS", "IMU_ACCEL_BW", "IMU_GYRO_FS", "IMU_GYRO_BW", "IMU_CALIB_INTERVAL", "IMU_CALIB_POINT_COUNT", "IMU_SAMPLING_FREQ", "LED1_CONFIG", "LED2_CONFIG", "LED3_CONFIG", "MP_ROLL_FILTER_CONSTANT", "MP_PITCH_FILTER_CONSTANT", "MP_THRESHOLD_X_ACCEL_LOW", "MP_THRESHOLD_X_ACCEL_HIGH", "MP_THRESHOLD_Y_ACCEL_LOW", "MP_THRESHOLD_Y_ACCEL_HIGH", "MP_THRESHOLD_Z_ACCEL_LOW", "MP_THRESHOLD_Z_ACCEL_HIGH", "MP_THRESHOLD_X_GYRO_LOW", "MP_THRESHOLD_X_GYRO_HIGH", "MP_THRESHOLD_Y_GYRO_LOW", "MP_THRESHOLD_Y_GYRO_HIGH", "MP_THRESHOLD_Z_GYRO_LOW", "MP_THRESHOLD_Z_GYRO_HIGH", "MP_THRESHOLD_ROLL_LOW", "MP_THRESHOLD_ROLL_HIGH", "MP_THRESHOLD_PITCH_LOW", "MP_THRESHOLD_PITCH_HIGH", "MP_THRESHOLD_YAW_LOW", "MP_THRESHOLD_YAW_HIGH", "MP_DETECTION_TYPE_X_ACCEL", "MP_DETECTION_TYPE_Y_ACCEL", "MP_DETECTION_TYPE_Z_ACCEL", "MP_DETECTION_TYPE_X_GYRO", "MP_DETECTION_TYPE_Y_GYRO", "MP_DETECTION_TYPE_Z_GYRO", "MP_DETECTION_TYPE_ROLL", "MP_DETECTION_TYPE_PITCH", "MP_DETECTION_TYPE_YAW"]
              n245 = property on="MD Thresholds Config.Get Parameter Index" class="DigNum (strict)"(error in=w629, "Val(Sgnl)"=w628) -> (error out=w632:errorcluster)  [unwired: 1 in, 1 out]
              n246 = case shown="1..18" w627 {
                selector: w627 -> [w635 _ _]
                tunnel: w632 -> [w642 w646 w654]
                tunnel: [w641 w645 w654] -> w631
                tunnel: w630 -> [w640 w644 _]
                tunnel: w626 -> [w636 w643 _]
                frame 1..18 {
                  n247 = Decrement(x=w635) -> (x-1=w633:u32)
                  n248 = Index Array(array=w636, index=w633) -> (element=w634:T15)
                  n249 = To Variant(anything=w634) -> (Variant=w637:variant)
                  n250 = Bundle By Name(cluster=T11 {"Data"=variant, "Command"=enum."UI_Event_Set_Config_RQST"} ("element"), "Data"=w637) -> (w638:T11)
                  n251 = Enqueue Element(queue=w640, element=w638, error in (no error)=w642) -> (error out=w641:errorcluster)  [unwired: 1 in, 2 out]
                }
                frame 19 {
                  n252 = for {
                    tunnel: w644 -> [w651]
                    shift-right: [w652] -> w645
                    shift-left: w646 -> [w653]
                    tunnel: w643 -> [w647] mode=indexing
                    n253 = To Variant(anything=w647) -> (Variant=w648:variant)
                    n254 = Bundle By Name(cluster=T11 {"Data"=variant, "Command"=enum."UI_Event_Set_Config_RQST"} ("element"), "Data"=w648) -> (w649:T11)
                    n255 = Enqueue Element(queue=w651, element=w649, error in (no error)=w653) -> (error out=w652:errorcluster)  [unwired: 1 in, 2 out]
                  }
                }
                frame Default {
                }
              }
            }
          }
        }
        frame "MD_TYPES_GET" {
          n256 = Unbundle By Name(w666) -> ("MPU_Stick_Queues.UI Event Handler"=w678:refnum<queue>)
          n257 = Unbundle By Name(w666) -> ("MD_Type_References.Get X accel threshold type"=w665:refnum<vi>, "MD_Type_References.Get Y accel threshold type"=w664:refnum<vi>, "MD_Type_References.Get Z accel threshold type"=w663:refnum<vi>, "MD_Type_References.Get X gyroscope threshold type"=w662:refnum<vi>, "MD_Type_References.Get Y gyroscope threshold type"=w661:refnum<vi>, "MD_Type_References.Get Z gyroscope threshold type"=w660:refnum<vi>, "MD_Type_References.Get roll threshold type"=w659:refnum<vi>, "MD_Type_References.Get pitch threshold type"=w658:refnum<vi>, "MD_Type_References.Get yaw threshold type"=w657:refnum<vi>, "MD_Type_References.Get all Motion detection type configurations"=w656:refnum<vi>)
          n258 = flat-sequence {
            tunnel: w676 -> [w681]
            tunnel: [w681] -> w675
            tunnel: [w680] -> w672
            frame #0 {
              n259 = local read "MD Types Config.Get Parameter Index"() -> (w680:u32)
            }
          }
          n260 = Build Array(w665, w664, w663, w662, w661, w660, w659, w658, w657, w656) -> (w655:refnum<vi>[])
          n261 = for {
            shift-right: [w685] -> w674
            shift-left: w675 -> [w686]
            tunnel: [w684] -> w671
            tunnel: [w683] -> w667
            tunnel: w655 -> [w682] mode=indexing
            i -> [w684]
            stop <- w683 stop-if-true
            n262 = property class="Bool (strict)"(reference=w682, error in=w686) -> (error out=w685:errorcluster, "Value"=w683:bool)  [unwired: 1 out]
          }
          n263 = Increment(x=w671) -> (x+1=w669:i32)
          n264 = Select(t=w669, s=w667, f=0) -> (s? t:f=w670:i32)
          n265 = To Unsigned Long Integer(number=w670) -> (unsigned 32bit integer=w673:u32)
          "MD Types Config.Get Parameter Index" <- w673
          n266 = Not Equal?(x=w673, y=w672) -> (x != y?=w679:bool)
          n267 = case shown="True" w679 {
            tunnel: [w687 w693] -> w677
            tunnel: w678 -> [_ w692]
            tunnel: w674 -> [w687 w691]
            tunnel: w673 -> [_ w690]
            tunnel: w672 -> [_ w689]
            frame False {
            }
            frame True {
              w688 = T15[] [enum."MP_DETECTION_TYPE_X_ACCEL", enum."MP_DETECTION_TYPE_Y_ACCEL", enum."MP_DETECTION_TYPE_Z_ACCEL", enum."MP_DETECTION_TYPE_X_GYRO", enum."MP_DETECTION_TYPE_Y_GYRO", enum."MP_DETECTION_TYPE_Z_GYRO", enum."MP_DETECTION_TYPE_ROLL", enum."MP_DETECTION_TYPE_PITCH", enum."MP_DETECTION_TYPE_YAW"] items=["IMU_ACCEL_FS", "IMU_ACCEL_BW", "IMU_GYRO_FS", "IMU_GYRO_BW", "IMU_CALIB_INTERVAL", "IMU_CALIB_POINT_COUNT", "IMU_SAMPLING_FREQ", "LED1_CONFIG", "LED2_CONFIG", "LED3_CONFIG", "MP_ROLL_FILTER_CONSTANT", "MP_PITCH_FILTER_CONSTANT", "MP_THRESHOLD_X_ACCEL_LOW", "MP_THRESHOLD_X_ACCEL_HIGH", "MP_THRESHOLD_Y_ACCEL_LOW", "MP_THRESHOLD_Y_ACCEL_HIGH", "MP_THRESHOLD_Z_ACCEL_LOW", "MP_THRESHOLD_Z_ACCEL_HIGH", "MP_THRESHOLD_X_GYRO_LOW", "MP_THRESHOLD_X_GYRO_HIGH", "MP_THRESHOLD_Y_GYRO_LOW", "MP_THRESHOLD_Y_GYRO_HIGH", "MP_THRESHOLD_Z_GYRO_LOW", "MP_THRESHOLD_Z_GYRO_HIGH", "MP_THRESHOLD_ROLL_LOW", "MP_THRESHOLD_ROLL_HIGH", "MP_THRESHOLD_PITCH_LOW", "MP_THRESHOLD_PITCH_HIGH", "MP_THRESHOLD_YAW_LOW", "MP_THRESHOLD_YAW_HIGH", "MP_DETECTION_TYPE_X_ACCEL", "MP_DETECTION_TYPE_Y_ACCEL", "MP_DETECTION_TYPE_Z_ACCEL", "MP_DETECTION_TYPE_X_GYRO", "MP_DETECTION_TYPE_Y_GYRO", "MP_DETECTION_TYPE_Z_GYRO", "MP_DETECTION_TYPE_ROLL", "MP_DETECTION_TYPE_PITCH", "MP_DETECTION_TYPE_YAW"]
              n268 = property on="MD Types Config.Get Parameter Index" class="DigNum (strict)"(error in=w691, "Val(Sgnl)"=w690) -> (error out=w694:errorcluster)  [unwired: 1 in, 1 out]
              n269 = case shown="1..9" w689 {
                selector: w689 -> [w697 _ _]
                tunnel: w694 -> [w704 w708 w716]
                tunnel: [w703 w707 w716] -> w693
                tunnel: w692 -> [w702 w706 _]
                tunnel: w688 -> [w698 w705 _]
                frame 1..9 {
                  n270 = Decrement(x=w697) -> (x-1=w695:u32)
                  n271 = Index Array(array=w698, index=w695) -> (element=w696:T15)
                  n272 = To Variant(anything=w696) -> (Variant=w699:variant)
                  n273 = Bundle By Name(cluster=T11 {"Data"=variant, "Command"=enum."UI_Event_Get_Config_RQST"} ("element"), "Data"=w699) -> (w700:T11)
                  n274 = Enqueue Element(queue=w702, element=w700, error in (no error)=w704) -> (error out=w703:errorcluster)  [unwired: 1 in, 2 out]
                }
                frame 10 {
                  n275 = for {
                    tunnel: w706 -> [w713]
                    shift-right: [w714] -> w707
                    shift-left: w708 -> [w715]
                    tunnel: w705 -> [w709] mode=indexing
                    n276 = To Variant(anything=w709) -> (Variant=w710:variant)
                    n277 = Bundle By Name(cluster=T11 {"Data"=variant, "Command"=enum."UI_Event_Get_Config_RQST"} ("element"), "Data"=w710) -> (w711:T11)
                    n278 = Enqueue Element(queue=w713, element=w711, error in (no error)=w715) -> (error out=w714:errorcluster)  [unwired: 1 in, 2 out]
                  }
                }
                frame Default {
                }
              }
            }
          }
        }
        frame "MD_TYPES_SET" {
          n279 = Unbundle By Name(w728) -> ("MPU_Stick_Queues.UI Event Handler"=w740:refnum<queue>)
          n280 = Unbundle By Name(w728) -> ("MD_Type_References.Set X accel threshold type"=w727:refnum<vi>, "MD_Type_References.Set Y accel threshold type"=w726:refnum<vi>, "MD_Type_References.Set Z accel threshold type"=w725:refnum<vi>, "MD_Type_References.Set X gyroscope threshold type"=w724:refnum<vi>, "MD_Type_References.Set Y gyroscope threshold type"=w723:refnum<vi>, "MD_Type_References.Set Z gyroscope threshold type"=w722:refnum<vi>, "MD_Type_References.Set roll threshold type"=w721:refnum<vi>, "MD_Type_References.Set pitch threshold type"=w720:refnum<vi>, "MD_Type_References.Set yaw threshold type"=w719:refnum<vi>, "MD_Type_References.Set all Motion detection type configurations"=w718:refnum<vi>)
          n281 = flat-sequence {
            tunnel: w738 -> [w743]
            tunnel: [w743] -> w737
            tunnel: [w742] -> w734
            frame #0 {
              n282 = local read "MD Types Config.Set Parameter Index"() -> (w742:u32)
            }
          }
          n283 = Build Array(w727, w726, w725, w724, w723, w722, w721, w720, w719, w718) -> (w717:refnum<vi>[])
          n284 = for {
            shift-right: [w747] -> w736
            shift-left: w737 -> [w748]
            tunnel: [w746] -> w733
            tunnel: [w745] -> w729
            tunnel: w717 -> [w744] mode=indexing
            i -> [w746]
            stop <- w745 stop-if-true
            n285 = property class="Bool (strict)"(reference=w744, error in=w748) -> (error out=w747:errorcluster, "Value"=w745:bool)  [unwired: 1 out]
          }
          n286 = Increment(x=w733) -> (x+1=w731:i32)
          n287 = Select(t=w731, s=w729, f=0) -> (s? t:f=w732:i32)
          n288 = To Unsigned Long Integer(number=w732) -> (unsigned 32bit integer=w735:u32)
          "MD Types Config.Set Parameter Index" <- w735
          n289 = Not Equal?(x=w735, y=w734) -> (x != y?=w741:bool)
          n290 = case shown="True" w741 {
            tunnel: [w749 w755] -> w739
            tunnel: w740 -> [_ w754]
            tunnel: w736 -> [w749 w753]
            tunnel: w735 -> [_ w752]
            tunnel: w734 -> [_ w751]
            frame False {
            }
            frame True {
              w750 = T15[] [enum."MP_DETECTION_TYPE_X_ACCEL", enum."MP_DETECTION_TYPE_Y_ACCEL", enum."MP_DETECTION_TYPE_Z_ACCEL", enum."MP_DETECTION_TYPE_X_GYRO", enum."MP_DETECTION_TYPE_Y_GYRO", enum."MP_DETECTION_TYPE_Z_GYRO", enum."MP_DETECTION_TYPE_ROLL", enum."MP_DETECTION_TYPE_PITCH", enum."MP_DETECTION_TYPE_YAW"] items=["IMU_ACCEL_FS", "IMU_ACCEL_BW", "IMU_GYRO_FS", "IMU_GYRO_BW", "IMU_CALIB_INTERVAL", "IMU_CALIB_POINT_COUNT", "IMU_SAMPLING_FREQ", "LED1_CONFIG", "LED2_CONFIG", "LED3_CONFIG", "MP_ROLL_FILTER_CONSTANT", "MP_PITCH_FILTER_CONSTANT", "MP_THRESHOLD_X_ACCEL_LOW", "MP_THRESHOLD_X_ACCEL_HIGH", "MP_THRESHOLD_Y_ACCEL_LOW", "MP_THRESHOLD_Y_ACCEL_HIGH", "MP_THRESHOLD_Z_ACCEL_LOW", "MP_THRESHOLD_Z_ACCEL_HIGH", "MP_THRESHOLD_X_GYRO_LOW", "MP_THRESHOLD_X_GYRO_HIGH", "MP_THRESHOLD_Y_GYRO_LOW", "MP_THRESHOLD_Y_GYRO_HIGH", "MP_THRESHOLD_Z_GYRO_LOW", "MP_THRESHOLD_Z_GYRO_HIGH", "MP_THRESHOLD_ROLL_LOW", "MP_THRESHOLD_ROLL_HIGH", "MP_THRESHOLD_PITCH_LOW", "MP_THRESHOLD_PITCH_HIGH", "MP_THRESHOLD_YAW_LOW", "MP_THRESHOLD_YAW_HIGH", "MP_DETECTION_TYPE_X_ACCEL", "MP_DETECTION_TYPE_Y_ACCEL", "MP_DETECTION_TYPE_Z_ACCEL", "MP_DETECTION_TYPE_X_GYRO", "MP_DETECTION_TYPE_Y_GYRO", "MP_DETECTION_TYPE_Z_GYRO", "MP_DETECTION_TYPE_ROLL", "MP_DETECTION_TYPE_PITCH", "MP_DETECTION_TYPE_YAW"]
              n291 = property on="MD Types Config.Set Parameter Index" class="DigNum (strict)"(error in=w753, "Val(Sgnl)"=w752) -> (error out=w756:errorcluster)  [unwired: 1 in, 1 out]
              n292 = case shown="1..9" w751 {
                selector: w751 -> [w759 _ _]
                tunnel: w756 -> [w766 w770 w778]
                tunnel: [w765 w769 w778] -> w755
                tunnel: w754 -> [w764 w768 _]
                tunnel: w750 -> [w760 w767 _]
                frame 1..9 {
                  n293 = Decrement(x=w759) -> (x-1=w757:u32)
                  n294 = Index Array(array=w760, index=w757) -> (element=w758:T15)
                  n295 = To Variant(anything=w758) -> (Variant=w761:variant)
                  n296 = Bundle By Name(cluster=T11 {"Data"=variant, "Command"=enum."UI_Event_Set_Config_RQST"} ("element"), "Data"=w761) -> (w762:T11)
                  n297 = Enqueue Element(queue=w764, element=w762, error in (no error)=w766) -> (error out=w765:errorcluster)  [unwired: 1 in, 2 out]
                }
                frame 10 {
                  n298 = for {
                    tunnel: w768 -> [w775]
                    shift-right: [w776] -> w769
                    shift-left: w770 -> [w777]
                    tunnel: w767 -> [w771] mode=indexing
                    n299 = To Variant(anything=w771) -> (Variant=w772:variant)
                    n300 = Bundle By Name(cluster=T11 {"Data"=variant, "Command"=enum."UI_Event_Set_Config_RQST"} ("element"), "Data"=w772) -> (w773:T11)
                    n301 = Enqueue Element(queue=w775, element=w773, error in (no error)=w777) -> (error out=w776:errorcluster)  [unwired: 1 in, 2 out]
                  }
                }
                frame Default {
                }
              }
            }
          }
        }
        frame "GRAPH_ADD_PARAMETER" {
          n302 = flat-sequence {
            tunnel: w789 -> [w821]
            tunnel: [w821] -> w788
            tunnel: [w820] -> w787
            frame #0 {
              n303 = local read "Primary.Add graph parameter"() -> (w820:bool)
            }
          }
          n304 = Unbundle By Name(w780) -> ("Primary_references.Add Parameter to Plot"=w790:refnum<vi>)
          n305 = Unbundle By Name(w780) -> ("Primary_references.Plot Parameter List"=w782:refnum<vi>)
          n306 = Unbundle By Name(w780) -> ("Primary_references.Parameter to monitor"=w781:refnum<vi>)
          n307 = property class="Bool (strict)"(reference=w790, error in=w788) -> (error out=w785:errorcluster, "Value"=w784:bool)  [unwired: 1 out]
          n308 = Not Equal?(x=w784, y=w787) -> (x != y?=w786:bool)
          n309 = Unbundle By Name(w780) -> ("MPU_Stick_Queues.Plot Updater"=w779:refnum<queue>)
          n310 = case shown="True" w786 {
            tunnel: w785 -> [w791 w807]
            tunnel: [w791 w796] -> w783
            tunnel: w784 -> [_ w806]
            tunnel: w782 -> [_ w805]
            tunnel: w781 -> [_ w803]
            tunnel: w779 -> [_ w792]
            frame False {
            }
            frame True {
              n311 = property class="Arr (strict)"(reference=w805) -> (reference out=w795:refnum<vi>, "Value"=w794:string[])  [unwired: 1 in, 1 out]
              n312 = property on="Primary.Add graph parameter" class="Bool (strict)"(error in=w807, "Val(Sgnl)"=w806) -> (error out=w804:errorcluster)  [unwired: 1 in, 1 out]
              n313 = property class="Enum (strict)"(reference=w803, error in=w804) -> (error out=w800:errorcluster, "Value"=w802:T1)  [unwired: 1 out]
              n314 = Index Array(array=string[] ["ACCEL_X", "ACCEL_Y", "ACCEL_Z", "GYRO_X", "GYRO_Y", "GYRO_Z", "ROLL_ACCEL", "ROLL_GYRO", "ROLL_COMP_FILTER", "PITCH_ACCEL", "PITCH_GYRO", "PITCH_COMP_FILTER", "YAW_ACCEL", "YAW_GYRO", "YAW_COMP_FILTER"] ("Strings []"), index=w802) -> (element=w793:string)
              n315 = Search 1D Array(1D array=w794, element=w793) -> (index of element=w799:i32)  [unwired: 1 in]
              n316 = Equal?(x=w799, y=-1) -> (x = y?=w797:bool)
              n317 = case shown="True" w797 {
                tunnel: w800 -> [w808 w816]
                tunnel: [w808 w813] -> w796
                tunnel: w795 -> [_ w819]
                tunnel: w794 -> [_ w818]
                tunnel: w793 -> [_ w811]
                tunnel: w792 -> [_ w814]
                frame False {
                }
                frame True {
                  n318 = Build Array (concatenate)(w818, w811) -> (w817:string[])
                  n319 = call "MPU_Stick_Plotter_Core.vi"("error in (no error)"=w816, "Channel Name"=w811, "Command"=MPU_Stick_Plotter_Core_Commands."Add Channel") -> ()  [unwired: 13 in, 4 out]
                  n320 = property class="Arr (strict)"(reference=w819, "Value"=w817) -> ()  [unwired: 1 in, 2 out]
                  n321 = To Variant(anything=w811) -> (Variant=w810:variant)
                  n322 = Bundle By Name(cluster=T11 {"Data"=variant, "Command"=enum."Plotter_Add_Channel"} ("element"), "Data"=w810) -> (w809:T11)
                  n323 = Enqueue Element At Opposite End(queue=w814, element=w809) -> (error out=w813:errorcluster)  [unwired: 2 in, 2 out]
                }
              }
            }
          }
        }
        frame "GRAPH_REMOVE_PARAMETER" {
          n324 = flat-sequence {
            tunnel: w831 -> [w860]
            tunnel: [w860] -> w830
            tunnel: [w859] -> w829
            frame #0 {
              n325 = local read "Primary.Remove graph parameter"() -> (w859:bool)
            }
          }
          n326 = Unbundle By Name(w822) -> ("Primary_references.Remove Parameter from Plot"=w832:refnum<vi>)
          n327 = Unbundle By Name(w822) -> ("Primary_references.Plot Parameter List"=w824:refnum<vi>)
          n328 = Unbundle By Name(w822) -> ("Primary_references.Parameter to monitor"=w823:refnum<vi>)
          n329 = property class="Bool (strict)"(reference=w832, error in=w830) -> (error out=w827:errorcluster, "Value"=w826:bool)  [unwired: 1 out]
          n330 = Not Equal?(x=w826, y=w829) -> (x != y?=w828:bool)
          n331 = case shown="True" w828 {
            tunnel: w827 -> [w833 w848]
            tunnel: [w833 w838] -> w825
            tunnel: w826 -> [_ w847]
            tunnel: w824 -> [_ w846]
            tunnel: w823 -> [_ w844]
            frame False {
            }
            frame True {
              n332 = property class="Arr (strict)"(reference=w846) -> (reference out=w837:refnum<vi>, "Value"=w836:string[])  [unwired: 1 in, 1 out]
              n333 = property on="Primary.Remove graph parameter" class="Bool (strict)"(error in=w848, "Val(Sgnl)"=w847) -> (error out=w845:errorcluster)  [unwired: 1 in, 1 out]
              n334 = property class="Enum (strict)"(reference=w844, error in=w845) -> (error out=w841:errorcluster, "Value"=w843:T1)  [unwired: 1 out]
              n335 = Index Array(array=string[] ["ACCEL_X", "ACCEL_Y", "ACCEL_Z", "GYRO_X", "GYRO_Y", "GYRO_Z", "ROLL_ACCEL", "ROLL_GYRO", "ROLL_COMP_FILTER", "PITCH_ACCEL", "PITCH_GYRO", "PITCH_COMP_FILTER", "YAW_ACCEL", "YAW_GYRO", "YAW_COMP_FILTER"] ("Strings []"), index=w843) -> (element=w835:string)
              n336 = Search 1D Array(1D array=w836, element=w835) -> (index of element=w834:i32)  [unwired: 1 in]
              n337 = Not Equal?(x=w834, y=-1) -> (x != y?=w839:bool)
              n338 = case shown="True" w839 {
                tunnel: w841 -> [w849 w857]
                tunnel: [w849 w856] -> w838
                tunnel: w837 -> [_ w858]
                tunnel: w836 -> [_ w853]
                tunnel: w835 -> [_ w855]
                tunnel: w834 -> [_ w852]
                frame False {
                }
                frame True {
                  n339 = Delete From Array(array=w853, length=1, index=w852) -> (array with subset deleted=w850:string[])  [unwired: 1 out]
                  n340 = call "MPU_Stick_Plotter_Core.vi"("error in (no error)"=w857, "Channel Name"=w855, "Command"=MPU_Stick_Plotter_Core_Commands."Remove Channel") -> ("error out"=w856:errorcluster)  [unwired: 13 in, 3 out]
                  n341 = property class="Arr (strict)"(reference=w858, "Value"=w850) -> ()  [unwired: 1 in, 2 out]
                }
              }
            }
          }
        }
        frame "SET_RANGE_AND_OFFSET" {
          n342 = flat-sequence {
            tunnel: w872 -> [w904]
            tunnel: [w904] -> w871
            tunnel: [w903] -> w870
            frame #0 {
              n343 = local read "Primary.Set Gain & Offset"() -> (w903:bool)
            }
          }
          n344 = Unbundle By Name(w863) -> ("Primary_references.Parameter to monitor"=w864:refnum<vi>)
          n345 = Unbundle By Name(w863) -> ("Primary_references.Set Range & Offset"=w873:refnum<vi>)
          n346 = Unbundle By Name(w863) -> ("Primary_references.Plot Parameter List"=w865:refnum<vi>, "Primary_references.Range"=w862:refnum<vi>, "Primary_references.Offset"=w861:refnum<vi>)
          n347 = property class="Bool (strict)"(reference=w873, error in=w871) -> (error out=w868:errorcluster, "Value"=w867:bool)  [unwired: 1 out]
          n348 = Not Equal?(x=w867, y=w870) -> (x != y?=w869:bool)
          n349 = case shown="True" w869 {
            tunnel: w868 -> [w874 w893]
            tunnel: [w874 w883] -> w866
            tunnel: w867 -> [_ w892]
            tunnel: w865 -> [_ w891]
            tunnel: w864 -> [_ w889]
            tunnel: w862 -> [_ w878]
            tunnel: w861 -> [_ w877]
            frame False {
            }
            frame True {
              n350 = property class="Arr (strict)"(reference=w891) -> (reference out=w882:refnum<vi>, "Value"=w881:string[])  [unwired: 1 in, 1 out]
              n351 = property on="Primary.Set Gain & Offset" class="Bool (strict)"(error in=w893, "Val(Sgnl)"=w892) -> (error out=w890:errorcluster)  [unwired: 1 in, 1 out]
              n352 = property class="DigNum (strict)"(reference=w878) -> ("Value"=w876:dbl)  [unwired: 1 in, 2 out]
              n353 = property class="DigNum (strict)"(reference=w877) -> ("Value"=w875:dbl)  [unwired: 1 in, 2 out]
              n354 = property class="Enum (strict)"(reference=w889, error in=w890) -> (error out=w886:errorcluster, "Value"=w888:T1)  [unwired: 1 out]
              n355 = Index Array(array=string[] ["ACCEL_X", "ACCEL_Y", "ACCEL_Z", "GYRO_X", "GYRO_Y", "GYRO_Z", "ROLL_ACCEL", "ROLL_GYRO", "ROLL_COMP_FILTER", "PITCH_ACCEL", "PITCH_GYRO", "PITCH_COMP_FILTER", "YAW_ACCEL", "YAW_GYRO", "YAW_COMP_FILTER"] ("Strings []"), index=w888) -> (element=w880:string)
              n356 = Search 1D Array(1D array=w881, element=w880) -> (index of element=w879:i32)  [unwired: 1 in]
              n357 = Not Equal?(x=w879, y=-1) -> (x != y?=w884:bool)
              n358 = case shown="True" w884 {
                tunnel: w886 -> [w894 w902]
                tunnel: [w894 w901] -> w883
                tunnel: w882 -> [_ _]
                tunnel: w880 -> [_ w900]
                tunnel: w879 -> [_ _]
                tunnel: w876 -> [_ w896]
                tunnel: w875 -> [_ w895]
                frame False {
                }
                frame True {
                  n359 = Bundle By Name(cluster=T14 {"Offset"=0.0, "Multiplier"=0.0} ("Offset & Multiplier"), "Multiplier"=w896, "Offset"=w895) -> (w897:T14)
                  n360 = call "MPU_Stick_Plotter_Core.vi"("Offset & Multiplier"=w897, "error in (no error)"=w902, "Channel Name"=w900, "Command"=MPU_Stick_Plotter_Core_Commands."Set Offset & Multiplier") -> ("error out"=w901:errorcluster)  [unwired: 12 in, 3 out]
                }
              }
            }
          }
        }
        frame "GET_RANGE_AND_OFFSET" {
          n361 = flat-sequence {
            tunnel: w916 -> [w947]
            tunnel: [w947] -> w915
            tunnel: [w946] -> w914
            frame #0 {
              n362 = local read "Primary.Get Gain & Offset"() -> (w946:bool)
            }
          }
          n363 = Unbundle By Name(w907) -> ("Primary_references.Parameter to monitor"=w908:refnum<vi>)
          n364 = Unbundle By Name(w907) -> ("Primary_references.Get Range & Offset"=w917:refnum<vi>)
          n365 = Unbundle By Name(w907) -> ("Primary_references.Plot Parameter List"=w909:refnum<vi>, "Primary_references.Range"=w906:refnum<vi>, "Primary_references.Offset"=w905:refnum<vi>)
          n366 = property class="Bool (strict)"(reference=w917, error in=w915) -> (error out=w912:errorcluster, "Value"=w911:bool)  [unwired: 1 out]
          n367 = Not Equal?(x=w911, y=w914) -> (x != y?=w913:bool)
          n368 = case shown="True" w913 {
            tunnel: w912 -> [w918 w935]
            tunnel: [w918 w925] -> w910
            tunnel: w911 -> [_ w934]
            tunnel: w909 -> [_ w933]
            tunnel: w908 -> [_ w931]
            tunnel: w906 -> [_ w920]
            tunnel: w905 -> [_ w919]
            frame False {
            }
            frame True {
              n369 = property class="Arr (strict)"(reference=w933) -> (reference out=w924:refnum<vi>, "Value"=w923:string[])  [unwired: 1 in, 1 out]
              n370 = property on="Primary.Get Gain & Offset" class="Bool (strict)"(error in=w935, "Val(Sgnl)"=w934) -> (error out=w932:errorcluster)  [unwired: 1 in, 1 out]
              n371 = property class="Enum (strict)"(reference=w931, error in=w932) -> (error out=w928:errorcluster, "Value"=w930:T1)  [unwired: 1 out]
              n372 = Index Array(array=string[] ["ACCEL_X", "ACCEL_Y", "ACCEL_Z", "GYRO_X", "GYRO_Y", "GYRO_Z", "ROLL_ACCEL", "ROLL_GYRO", "ROLL_COMP_FILTER", "PITCH_ACCEL", "PITCH_GYRO", "PITCH_COMP_FILTER", "YAW_ACCEL", "YAW_GYRO", "YAW_COMP_FILTER"] ("Strings []"), index=w930) -> (element=w922:string)
              n373 = Search 1D Array(1D array=w923, element=w922) -> (index of element=w921:i32)  [unwired: 1 in]
              n374 = Not Equal?(x=w921, y=-1) -> (x != y?=w926:bool)
              n375 = case shown="True" w926 {
                tunnel: w928 -> [w936 w945]
                tunnel: [w936 w944] -> w925
                tunnel: w924 -> [_ _]
                tunnel: w922 -> [_ w943]
                tunnel: w921 -> [_ _]
                tunnel: w920 -> [_ w940]
                tunnel: w919 -> [_ w938]
                frame False {
                }
                frame True {
                  n376 = call "MPU_Stick_Plotter_Core.vi"("error in (no error)"=w945, "Channel Name"=w943, "Command"=MPU_Stick_Plotter_Core_Commands."Get Offset & Multiplier") -> ("Plot Data"=w941:T16, "error out"=w944:errorcluster)  [unwired: 13 in, 2 out]
                  n377 = Unbundle By Name(w941) -> ("Range"=w939:dbl, "Offset"=w937:dbl)
                  n378 = property class="DigNum (strict)"(reference=w938, "Value"=w937) -> ()  [unwired: 1 in, 2 out]
                  n379 = property class="DigNum (strict)"(reference=w940, "Value"=w939) -> ()  [unwired: 1 in, 2 out]
                }
              }
            }
          }
        }
        frame "READ_RANGE_AND_OFFSET" {
          n380 = flat-sequence {
            tunnel: w960 -> [w990]
            tunnel: [w990] -> w952
            tunnel: [w989] -> w950
            frame #0 {
              n381 = local read "Primary.Parameter to monitor"() -> (w989:T1)
            }
          }
          n382 = Unbundle By Name(w956) -> ("Primary_references.Parameter to monitor"=w953:refnum<vi>)
          n383 = Unbundle By Name(w956) -> ("Primary_references.Parameter to monitor"=w957:refnum<vi>)
          n384 = Unbundle By Name(w956) -> ("Primary_references.Plot Parameter List"=w958:refnum<vi>, "Primary_references.Range"=w955:refnum<vi>, "Primary_references.Offset"=w954:refnum<vi>)
          n385 = property class="Enum (strict)"(reference=w953, error in=w952) -> (error out=w951:errorcluster, "Value"=w948:T1)  [unwired: 1 out]
          n386 = Not Equal?(x=w948, y=w950) -> (x != y?=w949:bool)
          n387 = case shown="True" w949 {
            tunnel: [w961 w971] -> w959
            tunnel: w958 -> [_ w978]
            tunnel: w957 -> [_ w977]
            tunnel: w955 -> [_ w966]
            tunnel: w954 -> [_ w965]
            tunnel: w951 -> [w961 w964]
            tunnel: w948 -> [_ w962]
            frame False {
            }
            frame True {
              n388 = property on="Primary.Parameter to monitor" class="Enum (strict)"(error in=w964, "Val(Sgnl)"=w962) -> (error out=w963:errorcluster)  [unwired: 1 in, 1 out]
              n389 = property class="Arr (strict)"(reference=w978) -> (reference out=w970:refnum<vi>, "Value"=w969:string[])  [unwired: 1 in, 1 out]
              n390 = property class="Enum (strict)"(reference=w977, error in=w963) -> (error out=w974:errorcluster, "Value"=w976:T1)  [unwired: 1 out]
              n391 = Index Array(array=string[] ["ACCEL_X", "ACCEL_Y", "ACCEL_Z", "GYRO_X", "GYRO_Y", "GYRO_Z", "ROLL_ACCEL", "ROLL_GYRO", "ROLL_COMP_FILTER", "PITCH_ACCEL", "PITCH_GYRO", "PITCH_COMP_FILTER", "YAW_ACCEL", "YAW_GYRO", "YAW_COMP_FILTER"] ("Strings []"), index=w976) -> (element=w968:string)
              n392 = Search 1D Array(1D array=w969, element=w968) -> (index of element=w967:i32)  [unwired: 1 in]
              n393 = Not Equal?(x=w967, y=-1) -> (x != y?=w972:bool)
              n394 = case shown="True" w972 {
                tunnel: w974 -> [w979 w988]
                tunnel: [w979 w987] -> w971
                tunnel: w970 -> [_ _]
                tunnel: w968 -> [_ w986]
                tunnel: w967 -> [_ _]
                tunnel: w966 -> [_ w983]
                tunnel: w965 -> [_ w981]
                frame False {
                }
                frame True {
                  n395 = call "MPU_Stick_Plotter_Core.vi"("error in (no error)"=w988, "Channel Name"=w986, "Command"=MPU_Stick_Plotter_Core_Commands."Get Offset & Multiplier") -> ("Plot Data"=w984:T16, "error out"=w987:errorcluster)  [unwired: 13 in, 2 out]
                  n396 = Unbundle By Name(w984) -> ("Range"=w982:dbl, "Offset"=w980:dbl)
                  n397 = property class="DigNum (strict)"(reference=w981, "Value"=w980) -> ()  [unwired: 1 in, 2 out]
                  n398 = property class="DigNum (strict)"(reference=w983, "Value"=w982) -> ()  [unwired: 1 in, 2 out]
                }
              }
            }
          }
        }
        frame "PLOT_PARAMETER_CHANGE" {
          n399 = flat-sequence {
            tunnel: w1004 -> [w1029]
            tunnel: [w1029] -> w996
            tunnel: [w1028] -> w994
            frame #0 {
              n400 = local read "Primary.Parameter to monitor A"() -> (w1028:T1)
            }
          }
          n401 = Unbundle By Name(w1000) -> ("Primary_references.Parameter to monitor"=w997:refnum<vi>)
          n402 = Unbundle By Name(w1000) -> ("Primary_references.Parameter to monitor"=w1001:refnum<vi>)
          n403 = Unbundle By Name(w1000) -> ("Primary_references.Parameter name"=w991:refnum<vi>, "Primary_references.Plot Parameter List"=w1002:refnum<vi>, "Primary_references.Range"=w999:refnum<vi>, "Primary_references.Offset"=w998:refnum<vi>)
          n404 = property class="Enum (strict)"(reference=w997, error in=w996) -> (error out=w995:errorcluster, "Value"=w992:T1)  [unwired: 1 out]
          n405 = Not Equal?(x=w992, y=w994) -> (x != y?=w993:bool)
          n406 = case shown="True" w993 {
            tunnel: [w1005 w1016] -> w1003
            tunnel: w1002 -> [_ w1023]
            tunnel: w1001 -> [_ w1022]
            tunnel: w999 -> [_ w1011]
            tunnel: w998 -> [_ w1010]
            tunnel: w995 -> [w1005 w1009]
            tunnel: w992 -> [_ w1007]
            tunnel: w991 -> [_ w1006]
            frame False {
            }
            frame True {
              n407 = property on="Primary.Parameter to monitor A" class="Enum (strict)"(error in=w1009, "Val(Sgnl)"=w1007) -> (error out=w1008:errorcluster)  [unwired: 1 in, 1 out]
              n408 = property class="Arr (strict)"(reference=w1023) -> (reference out=w1015:refnum<vi>, "Value"=w1014:string[])  [unwired: 1 in, 1 out]
              n409 = property class="Enum (strict)"(reference=w1022, error in=w1008) -> (error out=w1019:errorcluster, "Value"=w1021:T1)  [unwired: 1 out]
              n410 = Index Array(array=string[] ["ACCEL_X", "ACCEL_Y", "ACCEL_Z", "GYRO_X", "GYRO_Y", "GYRO_Z", "ROLL_ACCEL", "ROLL_GYRO", "ROLL_COMP_FILTER", "PITCH_ACCEL", "PITCH_GYRO", "PITCH_COMP_FILTER", "YAW_ACCEL", "YAW_GYRO", "YAW_COMP_FILTER"] ("Strings []"), index=w1021) -> (element=w1013:string)
              n411 = Search 1D Array(1D array=w1014, element=w1013) -> (index of element=w1012:i32)  [unwired: 1 in]
              n412 = Not Equal?(x=w1012, y=-1) -> (x != y?=w1017:bool)
              n413 = case shown="True" w1017 {
                tunnel: w1019 -> [w1024 w1027]
                tunnel: [w1024 w1027] -> w1016
                tunnel: w1015 -> [_ _]
                tunnel: w1013 -> [_ w1025]
                tunnel: w1012 -> [_ _]
                tunnel: w1011 -> [_ _]
                tunnel: w1010 -> [_ _]
                tunnel: w1006 -> [_ w1026]
                frame False {
                }
                frame True {
                  n414 = property class="Str"(reference=w1026, "Value"=w1025) -> ()  [unwired: 1 in, 2 out]
                }
              }
            }
          }
        }
        frame "UPDATE_PLOT_CURSOR_POSITION" {
          n415 = flat-sequence {
            tunnel: w1048 -> [w1077]
            tunnel: [w1077] -> w1044
            tunnel: [w1076] -> w1043
            frame #0 {
              n416 = local read "Primary.Cursor Position"() -> (w1076:T2)
            }
          }
          n417 = Unbundle By Name(w1045) -> ("Primary_references.Plot"=w1033:refnum<vi>)
          n418 = Unbundle By Name(w1045) -> ("Primary_references.Parameter to monitor"=w1046:refnum<vi>, "Primary_references.Plot Parameter List"=w1032:refnum<vi>)
          n419 = Unbundle By Name(w1045) -> ("Primary_references.Plot time (ms)"=w1031:refnum<vi>, "Primary_references.Plot value"=w1030:refnum<vi>)
          n420 = property class="XYGraph (strict)"(reference=w1033, error in=w1044) -> (error out=w1034:errorcluster, "Cursor.Cursor Position"=w1035:T2)  [unwired: 1 out]
          n421 = Unbundle By Name(w1043) -> ("X"=w1041:dbl, "Y"=w1039:dbl)
          n422 = Unbundle By Name(w1035) -> ("Cursor X"=w1042:dbl, "Cursor Y"=w1040:dbl)
          n423 = Not Equal?(x=w1042, y=w1041) -> (x != y?=w1038:bool)
          n424 = Not Equal?(x=w1040, y=w1039) -> (x != y?=w1037:bool)
          n425 = Or(x=w1038, y=w1037) -> (x .or. y?=w1036:bool)
          n426 = case shown="True" w1036 {
            tunnel: [w1049 w1060] -> w1047
            tunnel: w1046 -> [_ w1065]
            tunnel: w1035 -> [_ w1052]
            tunnel: w1034 -> [w1049 w1058]
            tunnel: w1032 -> [_ w1055]
            tunnel: w1031 -> [_ w1051]
            tunnel: w1030 -> [_ w1050]
            frame False {
            }
            frame True {
              n427 = property on="Primary.Cursor Position" class="Clust (strict)"(error in=w1058, "Val(Sgnl)"=w1052) -> (error out=w1057:errorcluster)  [unwired: 1 in, 1 out]
              n428 = property class="Arr (strict)"(reference=w1055) -> ("Value"=w1054:string[])  [unwired: 1 in, 2 out]
              n429 = property class="Enum (strict)"(reference=w1065, error in=w1057) -> (error out=w1063:errorcluster, "Value"=w1064:T1)  [unwired: 1 out]
              n430 = Index Array(array=string[] ["ACCEL_X", "ACCEL_Y", "ACCEL_Z", "GYRO_X", "GYRO_Y", "GYRO_Z", "ROLL_ACCEL", "ROLL_GYRO", "ROLL_COMP_FILTER", "PITCH_ACCEL", "PITCH_GYRO", "PITCH_COMP_FILTER", "YAW_ACCEL", "YAW_GYRO", "YAW_COMP_FILTER"] ("Strings []"), index=w1064) -> (element=w1053:string)
              n431 = Search 1D Array(1D array=w1054, element=w1053) -> (index of element=w1059:i32)  [unwired: 1 in]
              n432 = Not Equal?(x=w1059, y=-1) -> (x != y?=w1061:bool)
              n433 = case shown="True" w1061 {
                tunnel: w1063 -> [w1066 w1075]
                tunnel: [w1066 w1074] -> w1060
                tunnel: w1053 -> [_ w1073]
                tunnel: w1059 -> [_ _]
                tunnel: w1052 -> [_ w1071]
                tunnel: w1051 -> [_ w1070]
                tunnel: w1050 -> [_ w1069]
                frame False {
                }
                frame True {
                  n434 = call "MPU_Stick_Plotter_Core.vi"("Offset & Multiplier"=w1071, "error in (no error)"=w1075, "Channel Name"=w1073, "Command"=MPU_Stick_Plotter_Core_Commands."Get Cursor Data") -> ("Sample value"=w1068:dbl, "Sample time (ms)"=w1067:dbl, "error out"=w1074:errorcluster)  [unwired: 12 in, 1 out]
                  n435 = property class="DigNum (strict)"(reference=w1069, "Value"=w1068) -> ()  [unwired: 1 in, 2 out]
                  n436 = property class="DigNum (strict)"(reference=w1070, "Value"=w1067) -> ()  [unwired: 1 in, 2 out]
                }
              }
            }
          }
        }
        frame "CHANGE_RANGE_AND_OFFSET" {
          n437 = flat-sequence {
            tunnel: w1095 -> [w1127]
            tunnel: [w1127] -> w1088
            tunnel: [w1126] -> w1081
            tunnel: [w1125] -> w1080
            frame #0 {
              n438 = local read "Primary.Gain"() -> (w1126:dbl)
              n439 = local read "Primary.Offset"() -> (w1125:dbl)
            }
          }
          n440 = Unbundle By Name(w1091) -> ("Primary_references.Parameter to monitor"=w1092:refnum<vi>)
          n441 = Unbundle By Name(w1091) -> ("Primary_references.Plot Parameter List"=w1093:refnum<vi>, "Primary_references.Range"=w1090:refnum<vi>, "Primary_references.Offset"=w1089:refnum<vi>)
          n442 = Unbundle By Name(w1091) -> ("Primary_references.Range"=w1087:refnum<vi>, "Primary_references.Offset"=w1086:refnum<vi>)
          n443 = property class="DigNum (strict)"(reference=w1086) -> ("Value"=w1078:dbl)  [unwired: 1 in, 2 out]
          n444 = property class="DigNum (strict)"(reference=w1087, error in=w1088) -> (error out=w1082:errorcluster, "Value"=w1079:dbl)  [unwired: 1 out]
          n445 = Not Equal?(x=w1079, y=w1081) -> (x != y?=w1085:bool)
          n446 = Not Equal?(x=w1078, y=w1080) -> (x != y?=w1084:bool)
          n447 = Or(x=w1085, y=w1084) -> (x .or. y?=w1083:bool)
          n448 = case shown="True" w1083 {
            tunnel: [w1096 w1108] -> w1094
            tunnel: w1093 -> [_ w1115]
            tunnel: w1092 -> [_ w1114]
            tunnel: w1090 -> [_ w1103]
            tunnel: w1089 -> [_ w1102]
            tunnel: w1082 -> [w1096 w1101]
            tunnel: w1081 -> [_ _]
            tunnel: w1080 -> [_ _]
            tunnel: w1079 -> [_ w1098]
            tunnel: w1078 -> [_ w1097]
            frame False {
            }
            frame True {
              n449 = property on="Primary.Gain" class="DigNum (strict)"(error in=w1101, "Val(Sgnl)"=w1098) -> (error out=w1100:errorcluster)  [unwired: 1 in, 1 out]
              n450 = property class="Arr (strict)"(reference=w1115) -> (reference out=w1107:refnum<vi>, "Value"=w1106:string[])  [unwired: 1 in, 1 out]
              n451 = property on="Primary.Offset" class="DigNum (strict)"(error in=w1100, "Val(Sgnl)"=w1097) -> (error out=w1099:errorcluster)  [unwired: 1 in, 1 out]
              n452 = property class="Enum (strict)"(reference=w1114, error in=w1099) -> (error out=w1111:errorcluster, "Value"=w1113:T1)  [unwired: 1 out]
              n453 = Index Array(array=string[] ["ACCEL_X", "ACCEL_Y", "ACCEL_Z", "GYRO_X", "GYRO_Y", "GYRO_Z", "ROLL_ACCEL", "ROLL_GYRO", "ROLL_COMP_FILTER", "PITCH_ACCEL", "PITCH_GYRO", "PITCH_COMP_FILTER", "YAW_ACCEL", "YAW_GYRO", "YAW_COMP_FILTER"] ("Strings []"), index=w1113) -> (element=w1105:string)
              n454 = Search 1D Array(1D array=w1106, element=w1105) -> (index of element=w1104:i32)  [unwired: 1 in]
              n455 = Not Equal?(x=w1104, y=-1) -> (x != y?=w1109:bool)
              n456 = case shown="True" w1109 {
                tunnel: w1111 -> [w1116 w1124]
                tunnel: [w1116 w1123] -> w1108
                tunnel: w1107 -> [_ _]
                tunnel: w1105 -> [_ w1122]
                tunnel: w1104 -> [_ _]
                tunnel: w1103 -> [_ _]
                tunnel: w1102 -> [_ _]
                tunnel: w1098 -> [_ w1118]
                tunnel: w1097 -> [_ w1117]
                frame False {
                }
                frame True {
                  n457 = Bundle By Name(cluster=T14 {"Offset"=0.0, "Multiplier"=0.0} ("Offset & Multiplier"), "Multiplier"=w1118, "Offset"=w1117) -> (w1119:T14)
                  n458 = call "MPU_Stick_Plotter_Core.vi"("Offset & Multiplier"=w1119, "error in (no error)"=w1124, "Channel Name"=w1122, "Command"=MPU_Stick_Plotter_Core_Commands."Set Offset & Multiplier") -> ("error out"=w1123:errorcluster)  [unwired: 12 in, 3 out]
                }
              }
            }
          }
        }
      }
    }
    n459 = flat-sequence {
      tunnel: w7 -> [w16]
      tunnel: [w16] -> w6
      frame #0 {
        w15 = u32 100  # UI response time
        n460 = Wait (ms)(milliseconds to wait=w15) -> ()  [unwired: 1 out]
      }
    }
  }
  n461 = while {
    shift-right: [w1130] -> _
    shift-left: "MPU_Stick_Globals" -> [w1131]
    shift-right: [w1132] -> _
    shift-left: w1 -> [w1136]
    stop <- w1129 stop-if-true
    n462 = Unbundle By Name(w1131) -> ("MPU_Stick_Queues.UI Event Handler"=w1135:refnum<queue>)
    n463 = Dequeue Element(queue=w1135, error in (no error)=w1136) -> (element=w1128:T11, error out=w1134:errorcluster)  [unwired: 1 in, 2 out]
    n464 = Unbundle By Name(w1128) -> ("Command"=w1133:T12)
    n465 = case shown="\"UI_Event_Connect_Device_RQST\"" w1133 {
      tunnel: w1134 -> [w1139 w1145 w1198 w1219 w1240 w1286 w1336 w1364 w1399 w1419 w1444]
      tunnel: [w1139 w1144 w1170 w1222 w1246 w1292 w1331 w1360 w1396 w1415 w1435] -> w1132
      tunnel: w1131 -> [w1138 w1146 w1163 w1220 w1242 w1288 w1337 w1366 w1400 w1420 w1445]
      tunnel: [w1138 w1146 w1172 w1225 w1235 w1281 w1340 w1369 w1401 w1431 w1451] -> w1130
      tunnel: [FALSE TRUE FALSE FALSE FALSE FALSE FALSE FALSE FALSE FALSE FALSE] -> w1129
      tunnel: w1128 -> [_ _ _ _ _ _ _ _ _ w1429 w1449]
      frame Default {
      }
      frame "UI_Event_Exit_Application_RQST" {
        n466 = Unbundle By Name(w1146) -> ("MPU_Stick_Queues.3D View Updater"=w1140:refnum<queue>, "MPU_Stick_Queues.Plot Updater"=w1141:refnum<queue>, "MPU_Stick_Queues.Serial Port Reader"=w1142:refnum<queue>, "MPU_Stick_Queues.UI Indicators Updater"=w1143:refnum<queue>)
        n467 = disable-structure shown="Enabled" {
          disable-tunnel: w1145 -> [w1160 w1161]
          disable-tunnel: [w1156 w1161] -> w1144
          disable-tunnel: w1143 -> [w1155 _]
          disable-tunnel: w1142 -> [w1154 _]
          disable-tunnel: w1141 -> [w1153 _]
          disable-tunnel: w1140 -> [w1152 _]
          frame Disabled {
            n468 = Enqueue Element(queue=w1155, element=T11 {"Data"=variant, "Command"=enum."UI Indicators Exit"}, error in (no error)=w1160) -> (error out=w1159:errorcluster)  [unwired: 1 in, 2 out]
            n469 = Enqueue Element(queue=w1154, element=T11 {"Data"=variant, "Command"=enum."Read_Serial_Port_Data_Exit"}, error in (no error)=w1159) -> (error out=w1158:errorcluster)  [unwired: 1 in, 2 out]
            n470 = Enqueue Element(queue=w1153, element=T11 {"Data"=variant, "Command"=enum."Plotter_Exit"}, error in (no error)=w1158) -> (error out=w1157:errorcluster)  [unwired: 1 in, 2 out]
            n471 = Enqueue Element(queue=w1152, element=T11 {"Data"=variant, "Command"=enum."3D Viewer Exit"}, error in (no error)=w1157) -> (error out=w1156:errorcluster)  [unwired: 1 in, 2 out]
          }
          frame Enabled {
          }
        }
      }
      frame "UI_Event_Connect_Device_RQST" {
        w1174 = 0 ("Node ID")
        w1173 = u16 1000 ("Retry interval (ms)")
        n472 = Unbundle By Name(w1163) -> ("ADCP"=w1199:refnum<vi>)
        n473 = Unbundle By Name(w1163) -> ("Primary_references.Baud Rate"=w1194:refnum<vi>)
        n474 = Unbundle By Name(w1163) -> ("Primary_references.COM Port"=w1193:refnum<vi>)
        n475 = property class="LVClassControl (strict)"(reference=w1199) -> (reference out=w1188:refnum<vi>, error out=w1189:errorcluster, "Value"=w1197:refnum<class "ADCP.lvclass">)  [unwired: 1 in]
        n476 = property class="DigNum (strict)"(reference=w1194) -> ("Value"=w1192:u32)  [unwired: 1 in, 2 out]
        n477 = property class="VISAName"(reference=w1193) -> ("Value"=w1191:refnum<visa-resource-name>)  [unwired: 1 in, 2 out]
        n478 = Bundle By Name(cluster=T17 {"Symbol File Path"=path "", "Transmit Log File Path"=path "", "Receive Log File Path"=path "", "COM Port"="", "Baud rate"=0, "Number of retries"=0, "Retry interval (ms)"=0, "Session start time (ms)"=0, "Current time (ms)"=0, "Serialport timeout (ms)"=0} ("ADCP Session Parameters"), "Baud rate"=w1192, "COM Port"=w1191, "Number of retries"=u16 10, "Retry interval (ms)"=w1173, "Serialport timeout (ms)"=w1173) -> (w1195:T17)
        n479 = call <vilib>:"Application Directory.vi"() -> ("Application Directory"=w1183:path)
        n480 = Build Path(base path=w1183, name or relative path="MPU_Stick") -> (appended path=w1181:path)
        n481 = Build Path(base path=w1181, name or relative path="MPU_Stick.csv") -> (appended path=w1179:path)
        n482 = call "ADCP_Init_Session.vi"("error in (no error)"=w1198, "ADCP Session Parameters"=w1195, "ADCP in"=w1197) -> ("error out"=w1177:errorcluster, "ADCP out"=w1178:refnum<class "ADCP.lvclass">)  [unwired: 7 in]
        n483 = call "ADCP_Sync_Reset_Node_Connection.vi"("error in (no error)"=w1177, "Node ID"=w1174, "ADCP In"=w1178) -> ("error out"=w1175:errorcluster, "ADCP Out"=w1176:refnum<class "ADCP.lvclass">)  [unwired: 7 in]
        n484 = call "ADCP_Open_Node_Connection.vi"("error in (no error)"=w1175, "Node ID"=w1174, "ADCP In"=w1176) -> ("error out"=w1186:errorcluster, "ADCP Out"=w1185:refnum<class "ADCP.lvclass">)  [unwired: 7 in]
        n485 = call <vilib>:"Clear Errors.vi"("error in (no error)"=w1186) -> ("error out"=w1166:errorcluster)  [unwired: 5 in, 1 out]
        n486 = call "ADCP_read_symbol_file.vi"("error in (no error)"=w1166, "Symbol File Path"=w1179, "ADCP in"=w1185) -> ("error out"=w1167:errorcluster, "ADCP out"=w1184:refnum<class "ADCP.lvclass">)  [unwired: 5 in, 2 out]
        n487 = flat-sequence {
          tunnel: w1189 -> [w1213]
          tunnel: w1188 -> [w1212]
          tunnel: [w1211] -> w1187
          tunnel: w1184 -> [w1210]
          tunnel: w1167 -> [w1209]
          tunnel: [w1209] -> w1165
          frame #0 {
            n488 = property class="LVClassControl (strict)"(reference=w1212, error in=w1213, "Value"=w1210) -> (reference out=w1211:refnum<vi>)  [unwired: 1 out]
          }
        }
        n489 = Unbundle By Name(w1163) -> ("Primary_references.Plot"=w1162:refnum<vi>)
        n490 = disable-structure shown="Enabled" {
          disable-tunnel: w1165 -> [w1203 w1208]
          disable-tunnel: [w1202 w1208] -> w1164
          disable-tunnel: w1162 -> [w1201 _]
          frame Disabled {
            n491 = call "MPU_Stick_Plotter_Core.vi"("error in (no error)"=w1203, "Plot update interval (ms)"=u32 100, "Number of vertical divisions"=u16 10, "Plot reference"=w1201, "Command"=MPU_Stick_Plotter_Core_Commands."Reset", "Time axis length (ms)"=u32 20000) -> ("error out"=w1202:errorcluster)  [unwired: 10 in, 3 out]
          }
          frame Enabled {
          }
        }
        n492 = Bundle By Name(cluster=w1163, "ADCP"=w1187) -> (w1172:T3)
        n493 = flat-sequence {
          tunnel: w1164 -> [w1214]
          tunnel: [w1214] -> w1171
          frame #0 {
            n494 = global write "MPU_Stick_Read_Serial_Port_Emulator.vi" "Read Serial Port Emulator"(TRUE ("Read Serial Port Emulator")) -> ()
          }
        }
        n495 = Unbundle By Name(w1172) -> ("MPU_Stick_Queues.Serial Port Reader"=w1169:refnum<queue>)
        n496 = Enqueue Element(queue=w1169, element=T11 {"Data"=variant, "Command"=enum."Read_Serial_Port_Data_Continue"}, error in (no error)=w1171) -> (error out=w1170:errorcluster)  [unwired: 1 in, 2 out]
      }
      frame "UI_Event_Disconnect_Device_RQST" {
        n497 = Unbundle By Name(w1220) -> ("MPU_Stick_Queues.Serial Port Reader"=w1217:refnum<queue>)
        n498 = Unbundle By Name(w1220) -> ("ADCP"=w1229:refnum<vi>)
        n499 = property class="LVClassControl (strict)"(reference=w1229) -> (reference out=w1227:refnum<vi>, error out=w1228:errorcluster, "Value"=w1224:refnum<class "ADCP.lvclass">)  [unwired: 1 in]
        n500 = Enqueue Element(queue=w1217, element=T11 {"Data"=variant, "Command"=enum."Read_Serial_Port_Data_Pause"}, error in (no error)=w1219) -> (error out=w1218:errorcluster)  [unwired: 1 in, 2 out]
        n501 = call "ADCP_Close_Node_Connection.vi"("error in (no error)"=w1218, "Node ID"=0, "ADCP In"=w1224) -> ("error out"=w1222:errorcluster, "ADCP Out"=w1221:refnum<class "ADCP.lvclass">)  [unwired: 7 in]
        n502 = property class="LVClassControl (strict)"(reference=w1227, error in=w1228, "Value"=w1221) -> (reference out=w1226:refnum<vi>)  [unwired: 1 out]
        n503 = Bundle By Name(cluster=w1220, "ADCP"=w1226) -> (w1225:T3)
      }
      frame "UI_Event_Read_All_Configurations_RQST" {
        n504 = Unbundle By Name(w1242) -> ("ADCP"=w1241:refnum<vi>)
        n505 = property class="LVClassControl (strict)"(reference=w1241) -> (reference out=w1237:refnum<vi>, "Value"=w1238:refnum<class "ADCP.lvclass">)  [unwired: 1 in, 1 out]
        n506 = call "ADCP_Close_Node_Connection.vi"("error in (no error)"=w1240, "ADCP In"=w1238) -> ("error out"=w1239:errorcluster, "ADCP Out"=w1236:refnum<class "ADCP.lvclass">)  [unwired: 8 in]
        n507 = Unbundle By Name(w1242) -> ("MPU_Stick_Queues.Serial Port Reader"=w1244:refnum<queue>, "MPU_Stick_Queues.UI Event Handler"=w1243:refnum<queue>)
        n508 = property class="LVClassControl (strict)"(reference=w1237, "Value"=w1236) -> ()  [unwired: 1 in, 2 out]
        n509 = Enqueue Element(queue=w1244, element=T11 {"Data"=variant, "Command"=enum."Read_Serial_Port_Data_Pause"}, error in (no error)=w1239) -> (queue out=w1250:refnum<queue>, error out=w1251:errorcluster)  [unwired: 1 in, 1 out]
        n510 = while {
          tunnel: w1251 -> [w1270]
          tunnel: w1250 -> [_]
          tunnel: [w1268] -> w1249
          tunnel: w1243 -> [w1264]
          stop <- w1267 stop-if-true
          n511 = Dequeue Element(queue=w1264, error in (no error)=w1270) -> (element=w1269:T11, error out=w1268:errorcluster)  [unwired: 1 in, 2 out]
          n512 = Unbundle By Name(w1269) -> ("Command"=w1266:T12)
          n513 = Equal?(x=MPU_Stick_Queue_Commands."Read_Serial_Port_Data_Pause_ACK", y=w1266) -> (x = y?=w1267:bool)
        }
        n514 = for {
          N: 1 -> [_]
          shift-right: [w1275] -> w1247
          shift-left: w1249 -> [w1276]
          shift-right: [w1273] -> w1235
          shift-left: w1242 -> [w1274]
          i -> [w1271]
          n515 = call "MPU_Stick_Read_Write_Configuration.vi"("error in (no error)"=w1276, "Command"=MPU_Stick_Read_Write_Configurations_Command."Read All", "Configuration Parameter"=w1271, "MPU_Stick_Globals"=w1274) -> ("error out"=w1275:errorcluster, "MPU_Stick_Globals Out"=w1273:T3)  [unwired: 6 in]
        }
        n516 = Unbundle By Name(w1235) -> ("Primary_references.Connect Device"=w1248:refnum<vi>)
        n517 = property class="Bool (strict)"(reference=w1248) -> ("Value"=w1245:bool)  [unwired: 1 in, 2 out]
        n518 = Unbundle By Name(w1235) -> ("ADCP"=w1234:refnum<vi>)
        n519 = property class="LVClassControl (strict)"(reference=w1234) -> (reference out=w1232:refnum<vi>, "Value"=w1233:refnum<class "ADCP.lvclass">)  [unwired: 1 in, 1 out]
        n520 = case shown="True" w1245 {
          tunnel: w1247 -> [w1256 w1263]
          tunnel: [w1256 w1259] -> w1246
          tunnel: w1244 -> [_ w1262]
          tunnel: w1233 -> [w1255 w1258]
          tunnel: [w1255 w1257] -> w1231
          frame False {
          }
          frame True {
            n521 = Enqueue Element(queue=w1262, element=T11 {"Data"=variant, "Command"=enum."Read_Serial_Port_Data_Continue"}, error in (no error)=w1263) -> (error out=w1260:errorcluster)  [unwired: 1 in, 2 out]
            n522 = call "ADCP_Open_Node_Connection.vi"("error in (no error)"=w1260, "ADCP In"=w1258) -> ("error out"=w1259:errorcluster, "ADCP Out"=w1257:refnum<class "ADCP.lvclass">)  [unwired: 8 in]
          }
        }
        n523 = property class="LVClassControl (strict)"(reference=w1232, "Value"=w1231) -> ()  [unwired: 1 in, 2 out]
      }
      frame "UI_Event_Write_All_Configurations_RQST" {
        n524 = Unbundle By Name(w1288) -> ("ADCP"=w1287:refnum<vi>)
        n525 = property class="LVClassControl (strict)"(reference=w1287) -> (reference out=w1283:refnum<vi>, "Value"=w1285:refnum<class "ADCP.lvclass">)  [unwired: 1 in, 1 out]
        n526 = call "ADCP_Close_Node_Connection.vi"("error in (no error)"=w1286, "ADCP In"=w1285) -> ("error out"=w1284:errorcluster, "ADCP Out"=w1282:refnum<class "ADCP.lvclass">)  [unwired: 8 in]
        n527 = Unbundle By Name(w1288) -> ("MPU_Stick_Queues.Serial Port Reader"=w1290:refnum<queue>, "MPU_Stick_Queues.UI Event Handler"=w1289:refnum<queue>)
        n528 = property class="LVClassControl (strict)"(reference=w1283, "Value"=w1282) -> ()  [unwired: 1 in, 2 out]
        n529 = Enqueue Element(queue=w1290, element=T11 {"Data"=variant, "Command"=enum."Read_Serial_Port_Data_Pause"}, error in (no error)=w1284) -> (queue out=w1296:refnum<queue>, error out=w1297:errorcluster)  [unwired: 1 in, 1 out]
        n530 = while {
          tunnel: w1297 -> [w1316]
          tunnel: w1296 -> [_]
          tunnel: [w1314] -> w1295
          tunnel: w1289 -> [w1310]
          stop <- w1313 stop-if-true
          n531 = Dequeue Element(queue=w1310, error in (no error)=w1316) -> (element=w1315:T11, error out=w1314:errorcluster)  [unwired: 1 in, 2 out]
          n532 = Unbundle By Name(w1315) -> ("Command"=w1312:T12)
          n533 = Equal?(x=MPU_Stick_Queue_Commands."Read_Serial_Port_Data_Pause_ACK", y=w1312) -> (x = y?=w1313:bool)
        }
        n534 = for {
          N: 1 -> [_]
          shift-right: [w1321] -> w1293
          shift-left: w1295 -> [w1322]
          shift-right: [w1319] -> w1281
          shift-left: w1288 -> [w1320]
          i -> [w1317]
          n535 = call "MPU_Stick_Read_Write_Configuration.vi"("error in (no error)"=w1322, "Command"=MPU_Stick_Read_Write_Configurations_Command."Write All", "Configuration Parameter"=w1317, "MPU_Stick_Globals"=w1320) -> ("error out"=w1321:errorcluster, "MPU_Stick_Globals Out"=w1319:T3)  [unwired: 6 in]
        }
        n536 = Unbundle By Name(w1281) -> ("Primary_references.Connect Device"=w1294:refnum<vi>)
        n537 = Unbundle By Name(w1281) -> ("ADCP"=w1280:refnum<vi>)
        n538 = property class="LVClassControl (strict)"(reference=w1280) -> (reference out=w1278:refnum<vi>, "Value"=w1279:refnum<class "ADCP.lvclass">)  [unwired: 1 in, 1 out]
        n539 = property class="Bool (strict)"(reference=w1294) -> ("Value"=w1291:bool)  [unwired: 1 in, 2 out]
        n540 = case shown="True" w1291 {
          tunnel: w1293 -> [w1302 w1309]
          tunnel: [w1302 w1305] -> w1292
          tunnel: w1290 -> [_ w1308]
          tunnel: w1279 -> [w1301 w1304]
          tunnel: [w1301 w1303] -> w1277
          frame False {
          }
          frame True {
            n541 = Enqueue Element(queue=w1308, element=T11 {"Data"=variant, "Command"=enum."Read_Serial_Port_Data_Continue"}, error in (no error)=w1309) -> (error out=w1306:errorcluster)  [unwired: 1 in, 2 out]
            n542 = call "ADCP_Open_Node_Connection.vi"("error in (no error)"=w1306, "ADCP In"=w1304) -> ("error out"=w1305:errorcluster, "ADCP Out"=w1303:refnum<class "ADCP.lvclass">)  [unwired: 8 in]
          }
        }
        n543 = property class="LVClassControl (strict)"(reference=w1278, "Value"=w1277) -> ()  [unwired: 1 in, 2 out]
      }
      frame "UI_Event_Save_All_Configurations_RQST" {
        w1325 = "MPU_STICK:CONTROL:CONFIG_SAVE" ("Parameter Name")
        n544 = Unbundle By Name(w1337) -> ("MPU_Stick_Queues.UI Event Handler"=w1333:refnum<queue>, "MPU_Stick_Queues.Serial Port Reader"=w1330:refnum<queue>)
        n545 = Unbundle By Name(w1337) -> ("ADCP"=w1343:refnum<vi>)
        n546 = Enqueue Element(queue=w1330, element=T11 {"Data"=variant, "Command"=enum."Read_Serial_Port_Data_Pause"}, error in (no error)=w1336) -> (error out=w1334:errorcluster)  [unwired: 1 in, 2 out]
        n547 = while {
          tunnel: w1334 -> [w1351]
          tunnel: w1333 -> [w1350]
          tunnel: [w1345] -> w1332
          stop <- w1346 stop-if-true
          n548 = Dequeue Element(queue=w1350, error in (no error)=w1351) -> (element=w1349:T11, error out=w1345:errorcluster)  [unwired: 1 in, 2 out]
          n549 = Unbundle By Name(w1349) -> ("Command"=w1348:T12)
          n550 = Equal?(x=w1348, y=MPU_Stick_Queue_Commands."Read_Serial_Port_Data_Pause_ACK") -> (x = y?=w1346:bool)
        }
        n551 = property class="LVClassControl (strict)"(reference=w1343) -> (reference out=w1342:refnum<vi>, "Value"=w1339:refnum<class "ADCP.lvclass">)  [unwired: 1 in, 1 out]
        n552 = call "MPU_Stick_Write_General_Parameter.vi"("ADCP in"=w1339, "Parameter Name"=w1325, "Parameter Value"="1", "error out"=w1332) -> ("ADCP out"=w1327:refnum<class "ADCP.lvclass">, "error out"=w1328:errorcluster)  [unwired: 10 in]
        n553 = call "ADCP_write_parameter.vi"("ADCP in"=w1327, "Parameter Name"=w1325, "Parameter Value"="0", "error in (no error)"=w1328) -> ("ADCP out"=w1326:refnum<class "ADCP.lvclass">, "error out"=w1323:errorcluster)  [unwired: 9 in, 1 out]
        n554 = Enqueue Element(queue=w1330, element=T11 {"Data"=variant, "Command"=enum."Read_Serial_Port_Data_Continue"}, error in (no error)=w1323) -> (error out=w1331:errorcluster)  [unwired: 1 in, 2 out]
        n555 = property class="LVClassControl (strict)"(reference=w1342, "Value"=w1326) -> (reference out=w1341:refnum<vi>)  [unwired: 1 in, 1 out]
        n556 = Bundle By Name(cluster=w1337, "ADCP"=w1341) -> (w1340:T3)
      }
      frame "UI_Event_MP_Reset_RQST" {
        w1354 = "MPU_STICK:CONTROL:MP_RESET" ("Parameter Name")
        n557 = Unbundle By Name(w1366) -> ("ADCP"=w1372:refnum<vi>)
        n558 = Unbundle By Name(w1366) -> ("MPU_Stick_Queues.Serial Port Reader"=w1359:refnum<queue>, "MPU_Stick_Queues.UI Event Handler"=w1362:refnum<queue>)
        n559 = Enqueue Element(queue=w1359, element=T11 {"Data"=variant, "Command"=enum."Read_Serial_Port_Data_Pause"}, error in (no error)=w1364) -> (error out=w1363:errorcluster)  [unwired: 1 in, 2 out]
        n560 = while {
          tunnel: w1363 -> [w1380]
          tunnel: w1362 -> [w1379]
          tunnel: [w1375] -> w1361
          stop <- w1374 stop-if-true
          n561 = Dequeue Element(queue=w1379, error in (no error)=w1380) -> (element=w1378:T11, error out=w1375:errorcluster)  [unwired: 1 in, 2 out]
          n562 = Unbundle By Name(w1378) -> ("Command"=w1377:T12)
          n563 = Equal?(x=w1377, y=MPU_Stick_Queue_Commands."Read_Serial_Port_Data_Pause_ACK") -> (x = y?=w1374:bool)
        }
        n564 = property class="LVClassControl (strict)"(reference=w1372) -> (reference out=w1371:refnum<vi>, "Value"=w1368:refnum<class "ADCP.lvclass">)  [unwired: 1 in, 1 out]
        n565 = call "MPU_Stick_Write_General_Parameter.vi"("ADCP in"=w1368, "Parameter Name"=w1354, "Parameter Value"="1", "error out"=w1361) -> ("ADCP out"=w1357:refnum<class "ADCP.lvclass">, "error out"=w1356:errorcluster)  [unwired: 10 in]
        n566 = call "ADCP_write_parameter.vi"("ADCP in"=w1357, "Parameter Name"=w1354, "Parameter Value"="0", "error in (no error)"=w1356) -> ("ADCP out"=w1352:refnum<class "ADCP.lvclass">, "error out"=w1355:errorcluster)  [unwired: 9 in, 1 out]
        n567 = Enqueue Element(queue=w1359, element=T11 {"Data"=variant, "Command"=enum."Read_Serial_Port_Data_Continue"}, error in (no error)=w1355) -> (error out=w1360:errorcluster)  [unwired: 1 in, 2 out]
        n568 = property class="LVClassControl (strict)"(reference=w1371, "Value"=w1352) -> (reference out=w1370:refnum<vi>)  [unwired: 1 in, 1 out]
        n569 = Bundle By Name(cluster=w1366, "ADCP"=w1370) -> (w1369:T3)
      }
      frame "UI_Event_Calibrate_IMU_Sensor_RQST" {
        w1384 = "MPU_STICK:CONTROL:IMU_CALIBRATE" ("Parameter Name")
        n570 = Unbundle By Name(w1400) -> ("MPU_Stick_Queues.UI Event Handler"=w1387:refnum<queue>, "MPU_Stick_Queues.Serial Port Reader"=w1398:refnum<queue>)
        n571 = Unbundle By Name(w1400) -> ("ADCP"=w1404:refnum<vi>)
        n572 = Enqueue Element(queue=w1398, element=T11 {"Data"=variant, "Command"=enum."Read_Serial_Port_Data_Pause"}, error in (no error)=w1399) -> (queue out=w1395:refnum<queue>, error out=w1389:errorcluster)  [unwired: 1 in, 1 out]
        n573 = while {
          tunnel: w1389 -> [w1412]
          tunnel: [w1411] -> w1388
          tunnel: w1387 -> [w1410]
          stop <- w1407 stop-if-true
          n574 = Dequeue Element(queue=w1410, error in (no error)=w1412) -> (element=w1409:T11, error out=w1411:errorcluster)  [unwired: 1 in, 2 out]
          n575 = Unbundle By Name(w1409) -> ("Command"=w1408:T12)
          n576 = Equal?(x=w1408, y=MPU_Stick_Queue_Commands."Read_Serial_Port_Data_Pause_ACK") -> (x = y?=w1407:bool)
        }
        n577 = property class="LVClassControl (strict)"(reference=w1404) -> (reference out=w1403:refnum<vi>, "Value"=w1391:refnum<class "ADCP.lvclass">)  [unwired: 1 in, 1 out]
        n578 = call "ADCP_flush_serial_port.vi"("error in (no error)"=w1388, "ADCP In"=w1391) -> ("error out"=w1392:errorcluster, "ADCP Out"=w1390:refnum<class "ADCP.lvclass">)  [unwired: 8 in]
        n579 = call "MPU_Stick_Write_General_Parameter.vi"("ADCP in"=w1390, "Parameter Name"=w1384, "Parameter Value"="1", "error out"=w1392) -> ("ADCP out"=w1385:refnum<class "ADCP.lvclass">, "error out"=w1386:errorcluster)  [unwired: 10 in]
        n580 = call "ADCP_write_parameter.vi"("ADCP in"=w1385, "Parameter Name"=w1384, "Parameter Value"="0", "error in (no error)"=w1386) -> ("ADCP out"=w1381:refnum<class "ADCP.lvclass">, "error out"=w1382:errorcluster)  [unwired: 9 in, 1 out]
        n581 = Enqueue Element(queue=w1395, element=T11 {"Data"=variant, "Command"=enum."Read_Serial_Port_Data_Continue"}, error in (no error)=w1382) -> (error out=w1396:errorcluster)  [unwired: 1 in, 2 out]
        n582 = property class="LVClassControl (strict)"(reference=w1403, "Value"=w1381) -> (reference out=w1402:refnum<vi>)  [unwired: 1 in, 1 out]
        n583 = Bundle By Name(cluster=w1400, "ADCP"=w1402) -> (w1401:T3)
      }
      frame "UI_Event_Get_Config_RQST" {
        n584 = Unbundle By Name(w1429) -> ("Data"=w1428:variant)
        n585 = Unbundle By Name(w1420) -> ("MPU_Stick_Queues.Serial Port Reader"=w1414:refnum<queue>)
        n586 = Variant To Data(type=MPU_Stick_Config_Parameters."IMU_ACCEL_FS" ("Enum"), Variant=w1428) -> (data=w1426:T15)  [unwired: 1 in, 1 out]
        n587 = Enqueue Element(queue=w1414, element=T11 {"Data"=variant, "Command"=enum."Read_Serial_Port_Data_Pause"}, error in (no error)=w1419) -> (error out=w1418:errorcluster)  [unwired: 1 in, 2 out]
        n588 = Unbundle By Name(w1420) -> ("ADCP"=w1424:refnum<vi>)
        n589 = property class="LVClassControl (strict)"(reference=w1424) -> (reference out=w1422:refnum<vi>, "Value"=w1423:refnum<class "ADCP.lvclass">)  [unwired: 1 in, 1 out]
        n590 = call "ADCP_flush_serial_port.vi"("error in (no error)"=w1418, "ADCP In"=w1423) -> ("error out"=w1425:errorcluster, "ADCP Out"=w1421:refnum<class "ADCP.lvclass">)  [unwired: 8 in]
        n591 = property class="LVClassControl (strict)"(reference=w1422, "Value"=w1421) -> ()  [unwired: 1 in, 2 out]
        n592 = call "MPU_Stick_Read_Write_Configuration.vi"("error in (no error)"=w1425, "Command"=MPU_Stick_Read_Write_Configurations_Command."Read", "Configuration Parameter"=w1426, "MPU_Stick_Globals"=w1420) -> ("error out"=w1416:errorcluster, "MPU_Stick_Globals Out"=w1431:T3)  [unwired: 6 in]
        n593 = Enqueue Element(queue=w1414, element=T11 {"Data"=variant, "Command"=enum."Read_Serial_Port_Data_Continue"}, error in (no error)=w1416) -> (error out=w1415:errorcluster)  [unwired: 1 in, 2 out]
      }
      frame "UI_Event_Set_Config_RQST" {
        n594 = Unbundle By Name(w1449) -> ("Data"=w1448:variant)
        n595 = Unbundle By Name(w1445) -> ("MPU_Stick_Queues.Serial Port Reader"=w1434:refnum<queue>, "ADCP"=w1441:refnum<vi>)
        n596 = Variant To Data(type=MPU_Stick_Config_Parameters."IMU_ACCEL_FS" ("Enum"), Variant=w1448) -> (data=w1446:T15)  [unwired: 1 in, 1 out]
        n597 = property class="LVClassControl (strict)"(reference=w1441) -> (reference out=w1439:refnum<vi>, "Value"=w1440:refnum<class "ADCP.lvclass">)  [unwired: 1 in, 1 out]
        n598 = Enqueue Element(queue=w1434, element=T11 {"Data"=variant, "Command"=enum."Read_Serial_Port_Data_Pause"}, error in (no error)=w1444) -> (error out=w1442:errorcluster)  [unwired: 1 in, 2 out]
        n599 = call "ADCP_flush_serial_port.vi"("error in (no error)"=w1442, "ADCP In"=w1440) -> ("error out"=w1437:errorcluster, "ADCP Out"=w1438:refnum<class "ADCP.lvclass">)  [unwired: 8 in]
        n600 = property class="LVClassControl (strict)"(reference=w1439, "Value"=w1438) -> ()  [unwired: 1 in, 2 out]
        n601 = call "MPU_Stick_Read_Write_Configuration.vi"("error in (no error)"=w1437, "Command"=MPU_Stick_Read_Write_Configurations_Command."Write", "Configuration Parameter"=w1446, "MPU_Stick_Globals"=w1445) -> ("error out"=w1436:errorcluster, "MPU_Stick_Globals Out"=w1451:T3)  [unwired: 6 in]
        n602 = Enqueue Element(queue=w1434, element=T11 {"Data"=variant, "Command"=enum."Read_Serial_Port_Data_Continue"}, error in (no error)=w1436) -> (error out=w1435:errorcluster)  [unwired: 1 in, 2 out]
      }
    }
  }
